vi "LabscanV1.vi"() -> ()   [LabVIEW 2019]
doc: "Ce Vi est le programme principale du système de spectroscopie pompe-sonde. Il permet d'effectuer des séries de mesures où l'on fait varier le délais entre un faisceaux d'excitation dit pompe et un faisceaux de mesure dit sonde, et où l'on mesure l'interaction des deux faisceaux en coupant momentanément le faisceau pompe. Le programme coordonne la ligne à délai, le shutter de la pompe et effectue l'acquisition de donnée. Les données sont affichées sur la fenêtres graphiques et on peut les sauvegarder dans un fichier texte. De multiple options sont disponible pour modifier les paramètres d'exécutions des balayages. Le programme facilite ainsi les mesures expérimentales."
uses:
  Experiment Class/Experiment.lvclass
  Interface Class/Interface.lvclass
  DevicesClass/BaseDevice/BaseDevice.lvclass
  <vilib>/Utility/miscctls.llb/LVPointTypeDef.ctl
  <vilib>/Utility/error.llb/DialogType.ctl
  <vilib>/event_ctls.llb/sizeaction.ctl
  <vilib>/event_ctls.llb/panelstate.ctl
  Interface Class/PlotChange.ctl
  <userlib>/GenProg/SetCtrlPropGen.vi
  Interface Class/Accessor/SetExperimentClass.vi
  <vilib>/Platform/browser.llb/Open URL in Default Browser (path).vi
  <userlib>/GenProg/SetCtrlPropGenSgl.vi
  DevicesClass/InstrumentsClass/MultiHarp150/MultiHarp150.lvclass
  DevicesClass/InstrumentsClass/AttoAMC/AttoAMC.lvclass
  DevicesClass/InstrumentsClass/TaikoLaser/TaikoLaser.lvclass
  DevicesClass/InstrumentsClass/ThorPM100A/ThorPM100A.lvclass
  DevicesClass/InstrumentsClass/AppliedMotionDrive/AppliedMotionDrive.lvclass
  DevicesClass/InstrumentsClass/ESP301/ESP301.lvclass
  DevicesClass/InstrumentsClass/AndorSpectro/AndorSpectro.lvclass
panel:
  in  "Load startup Exp.":bool=TRUE
  in  "Discard":bool
  in  "refresh test":bool
  out "Experiment Path":path
  out "queue out":refnum<queue>
  out "user event out":refnum<user-event>
  out "WrtGrpDel":u32
  out "WrtDatDel":u32
  in  "BaseDevice.lvclass":refnum<class "BaseDevice.lvclass">
  out "sem1":T1
  in  "DataFileRef":refnum<file>
  out "Exper.lvclass":refnum<class "Experiment.lvclass">
  out "ErrorOutAcq":errorcluster
  in  "HdrFileName":path
  out "error out":errorcluster
  in  "Error in":errorcluster
  out "ScanList":string[](array[string])
  in  "AcqEnd":bool caption="Fin Balayage"
  out "AcqComp":bool
  in  "Pause":bool
  in  "AcqStop":bool caption="Arrêt Balayage"
  out "Graph_VIs":refnum<vi>[](array[refnum])
  out "Graph_FA":refnum<vi>[](array[refnum])
  in  "stop":bool
  in  "Interface.lvclass":refnum<class "Interface.lvclass">
  in  "CtrlsTab":enum32{"Balayage", "Experiment", "Tracés"}(tab)
  in  "Single Par":bool caption="Single Parameter"
  in  "Scan Function":u16(ring) items=["Scan Pos (Arb)@Tools", "Indice de Point (Points)@Tools", "Scan Pos (Arb)@Tools_2", "Scan Pos (Arb)@Tools_3"]
  in  "path":path caption="Chemin du fichier de Sauvegarde"
  in  "Ouvrir":bool
  out "Temps Balayage":dbl format="%<%H:%M:%S>t"
  in  "DescKword":string caption="Description Keyword"
  in  "ScanFunc":string(tree) caption="Scan Functions"
  in  "MeasFunc":i32(listbox) caption="Measurements Instruments"
  out "MeasTime":u32 caption="Last Meas. Time (ms, all devices)"
  out "AvgPointTime(ms)":u32
  out "MeasTimes":u32[](array[numeric]) caption="Measurement Times (ms, by device)"
  out "ScanTimes":u32[](array[numeric]) caption="Scan Times (ms, by device)"
  in  "nb pos":i32 caption="Total Scan Points"
  out "Points Left":u32
  in  "Listbox":i32[](listbox)=[0] caption="Affichage des courbes"
  in  "Acq":bool caption="Balayage"
  # "Variables internes Balayages"
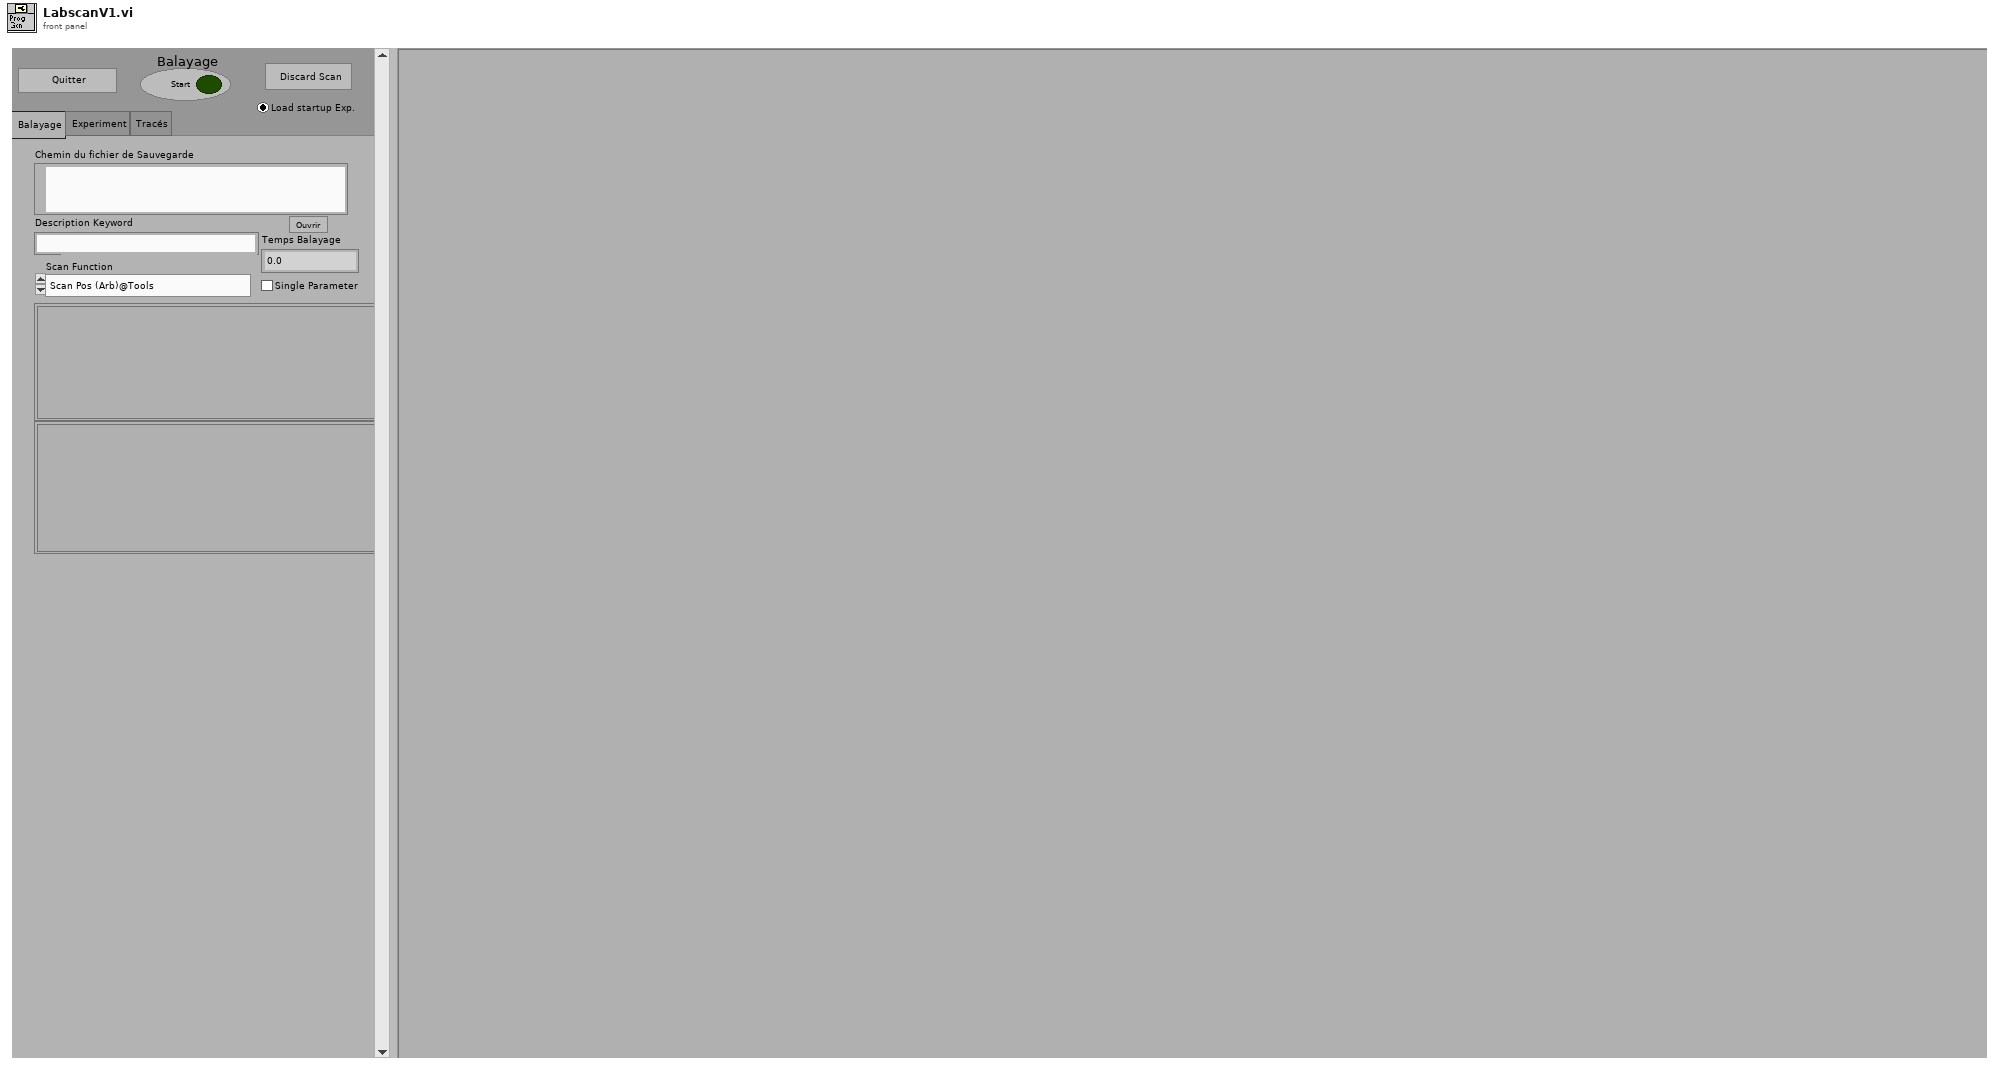
[diagram p1: front panel]
types:
  T1 = typedef "Semaphore RefNum" = refnum<k1>
  T2 = enum16{"Enable", "Disable", "DisAndGrayed", "ReinitToDefVal", "EnumElementsArr"}
  T3 = typedef "LVPointTypeDef.ctl" = cluster{"Horizontal":i16, "Vertical":i16}
  T4 = enum32{"Invalid", "Standard", "Closed", "Hidden", "Minimized", "Maximized"}
  T5 = enum16{"Répertoire du VI actuel", "Répertoire du parent 1", "Répertoire du parent 2", "Répertoire du parent 3"}
  T6 = enum16{"Text", "Background", "Item Symbol", "Open/Close Symbol", "Hierarchy Lines", "Right Border", "Bottom Border", "Bottom Right Corner", "Unknown Part"}
  T7 = typedef "panelstate.ctl" = enum32{"Standard", "Minimized", "Maximized"}
  T8 = typedef "sizeaction.ctl" = enum32{"Minimized", "Maximized", "Resized"}
  T9 = cluster{"Message":string, "Data":variant, "Code":i32}
  T10 = enum16{"No Item Sel", "One Item Sel", "Many Items Sel"}
  T11 = typedef "PlotChange.ctl" = cluster{"PlotIdx":i32, "PlotAttrib":cluster{"Color":u32, "PointStyle":u8, "LineStyle":u8, "Interp":u8, "LineWidth":u8, "BarPlotStyle":u8, "FillTo":i16, "XScaleIdx":u32, "YScaleIdx":u32, "Anti-Aliased":bool, "LabelFormat":u8, "TransitionType":u8, "TransitionLocation":u8, "DigitalLineStyle":u8}, "GraphId":i32, "Crv Visible":bool}
  T12 = cluster{dbl[], "XparInstrInd":i32, "YparInstrInd":i32}
  T13 = typedef "LVPositionTypeDef.ctl" = cluster{"Left":i32, "Top":i32}
  T14 = typedef "LVRectTypeDef.ctl" = cluster{"Left":i16, "Top":i16, "Right":i16, "Bottom":i16}
  T15 = typedef "DialogType.ctl" = u16
  T16 = typedef "Interface.lvclass/CurveSetup.ctl" = cluster{"CurveName":string, "YParam":string, "XParam":string, "ZParam ":string, "GroupName":string, "LinWdth":u8, "PntCol":u32, "LinCol":u32, "LablFor":u8, "XScale":u32, "YScale":u32, "Interpol":u8, "DisplayName":string, "FillType":i16, "LineStyle":u8, "PntStyle":u8, "BarTyp":u8, "GraphIndex":i32, "Visible":bool, "XScaleName":string, "YScaleName":string, "XYGraph_Ref":refnum<vi>, "Data Only":bool, "DataQ Ref":refnum<queue>, "XParQ Ref":refnum<queue>, "XParamInd":i32, "ScanInd":i32, "File Path":path}
  T17 = typedef "ArrDevData.ctl" = cluster{"MeasDatOut":dbl[][], "XDatOut":dbl[][], "YDatOut":dbl[][], "DevID":i32}
  T18 = enum16{"Left Button", "Center Button", "Right Button", "Window Close"}
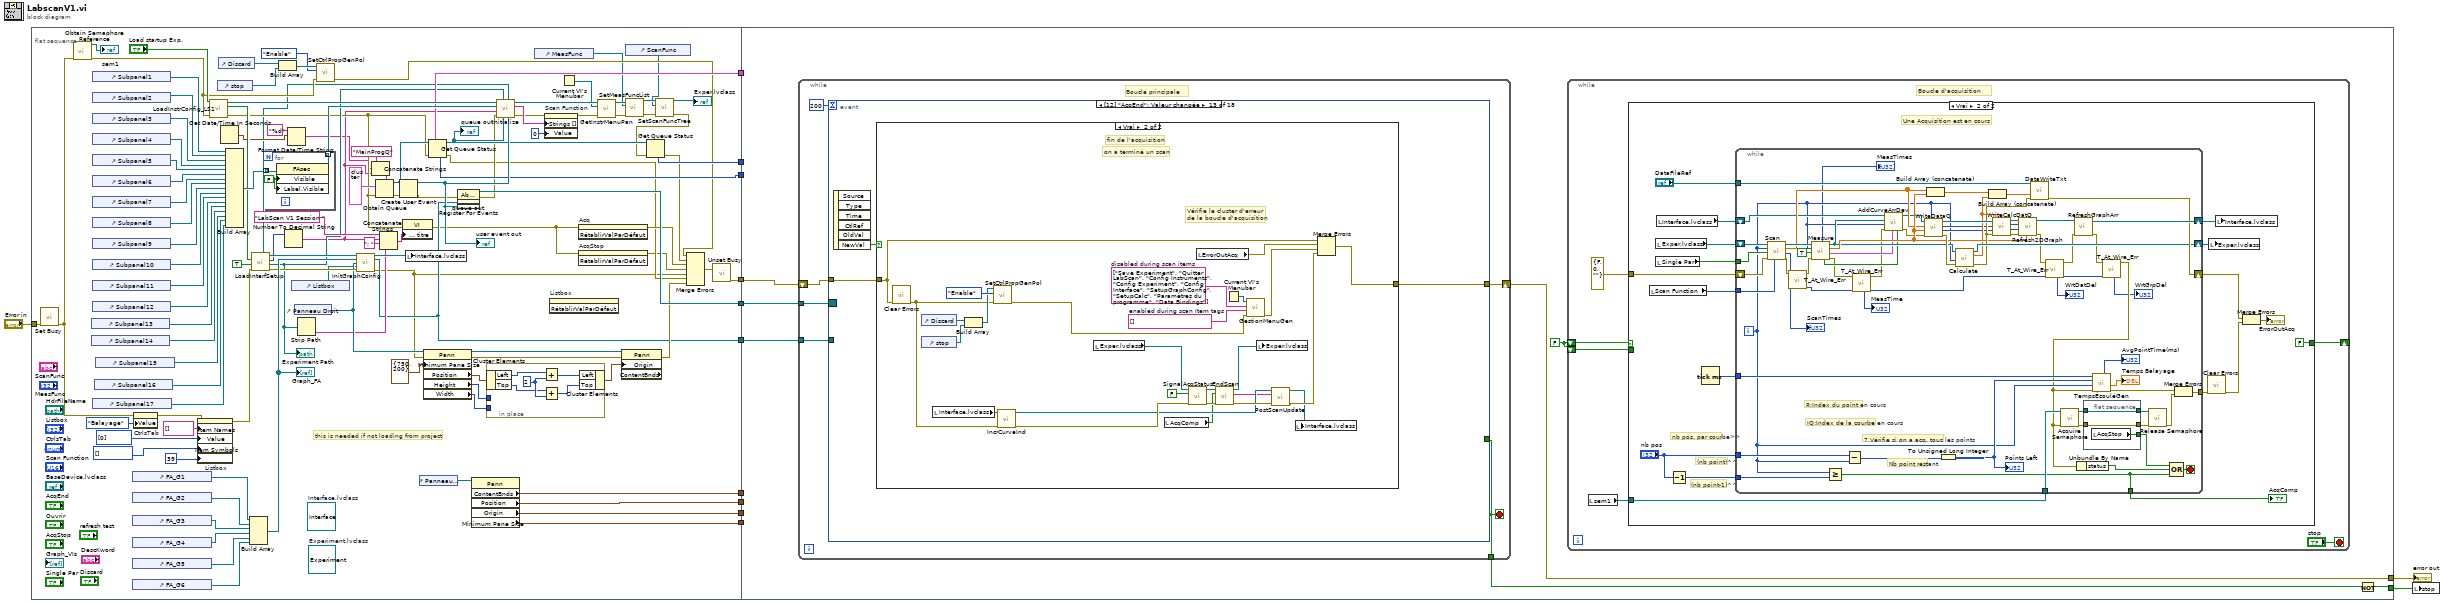
[diagram p0: block diagram]
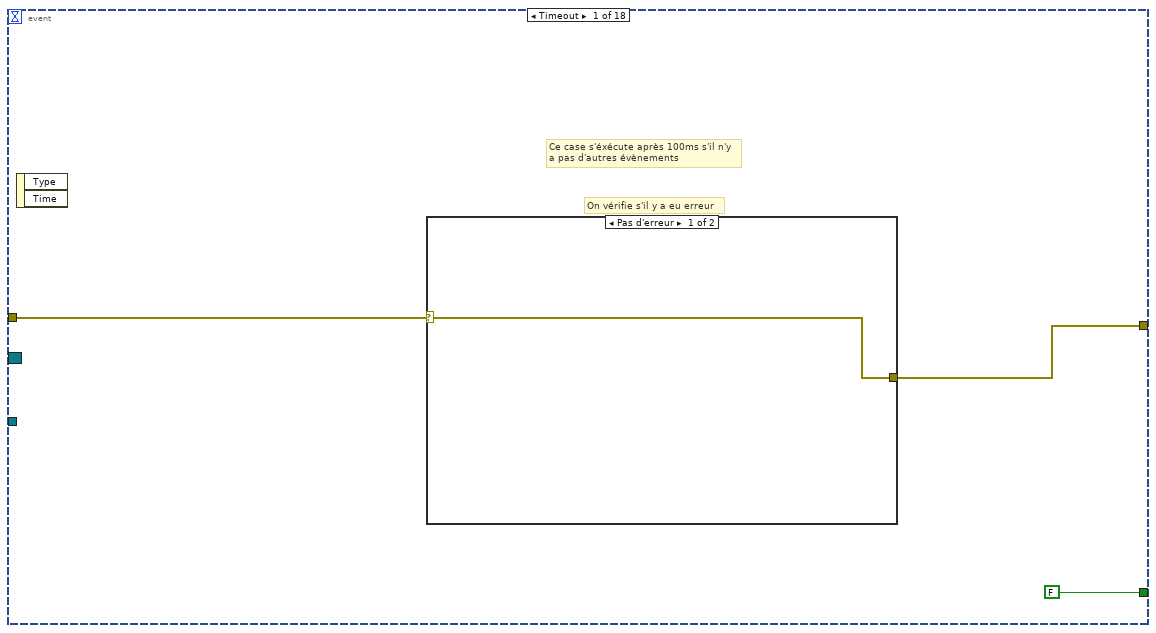
[diagram p2: hidden frame]
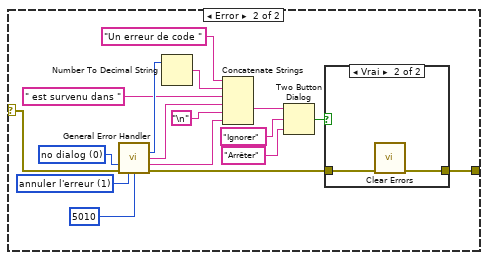
[diagram p3: hidden frame]
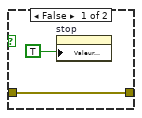
[diagram p4: hidden frame]
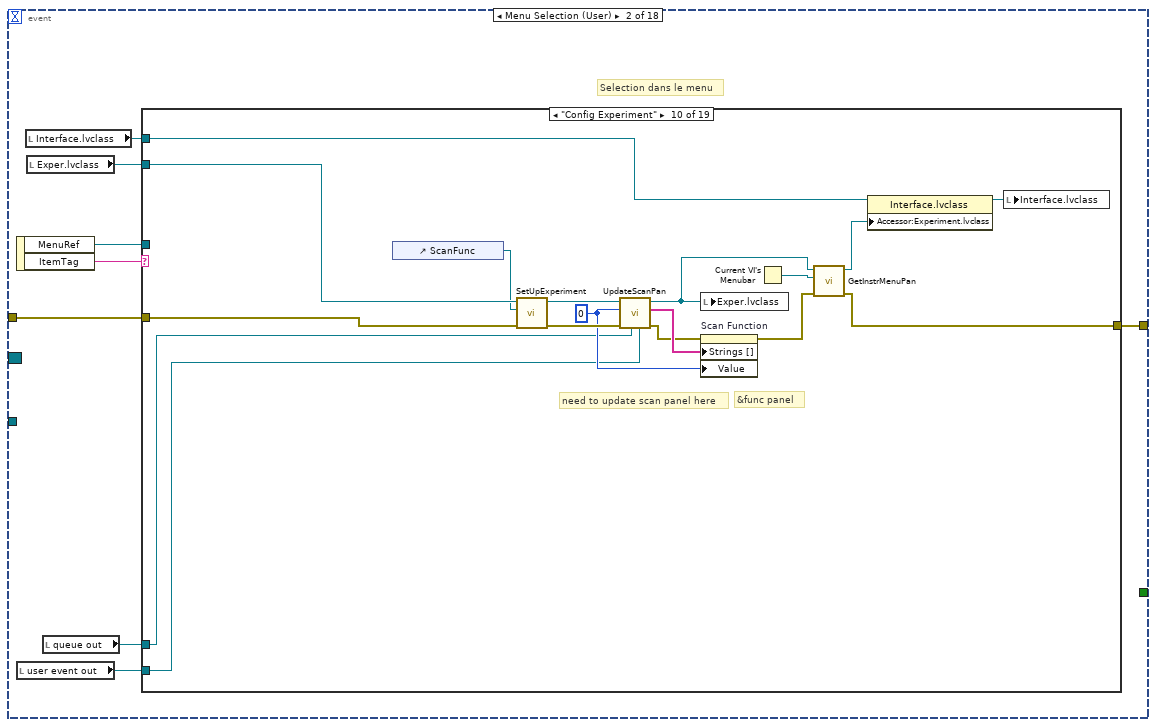
[diagram p5: hidden frame]
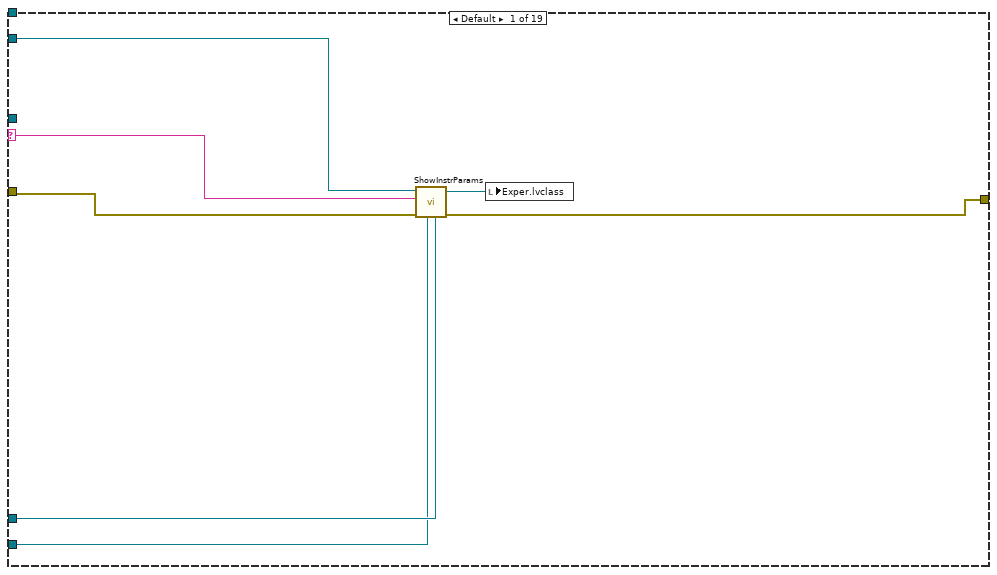
[diagram p6: hidden frame]
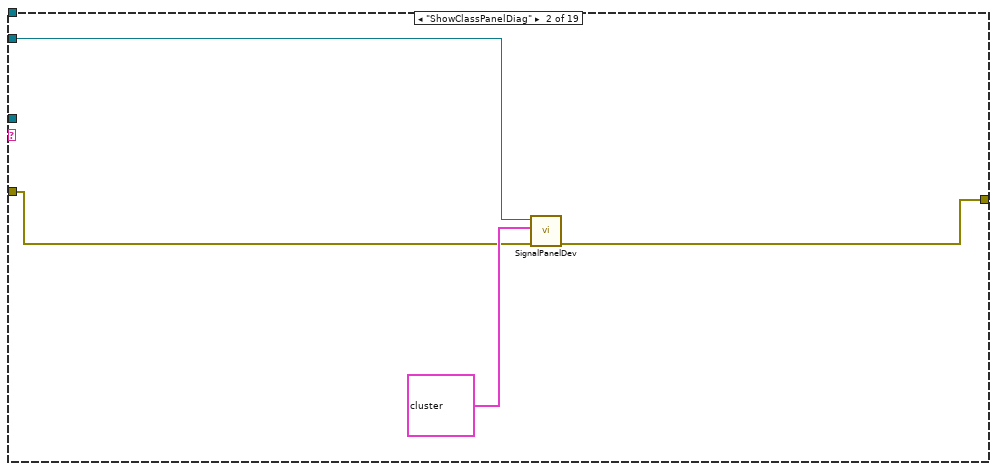
[diagram p7: hidden frame]
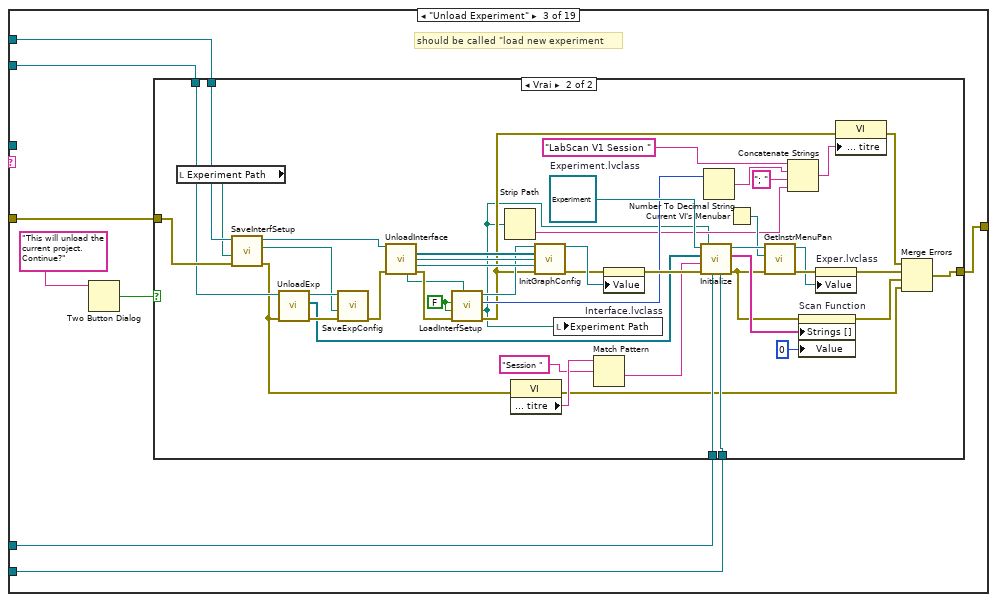
[diagram p8: hidden frame]
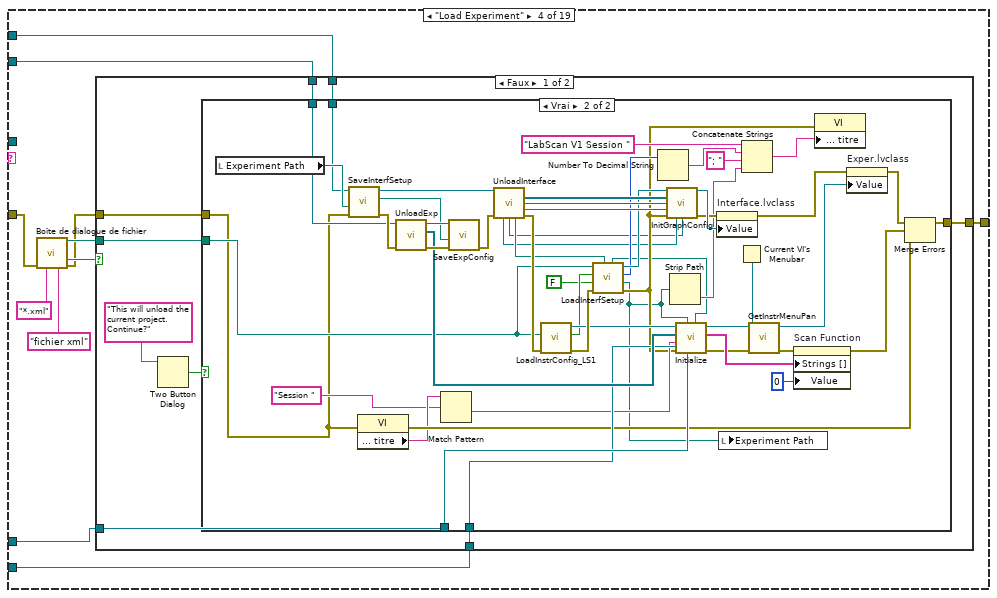
[diagram p10: hidden frame]
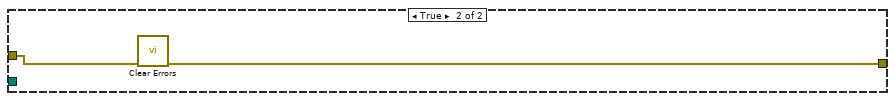
[diagram p12: hidden frame]
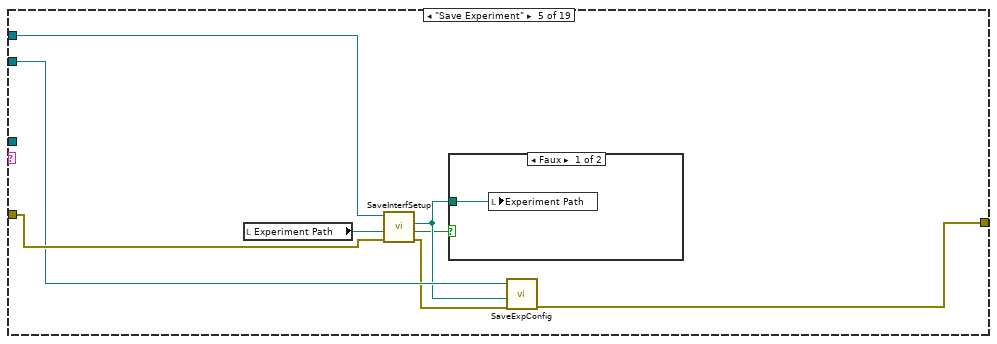
[diagram p13: hidden frame]
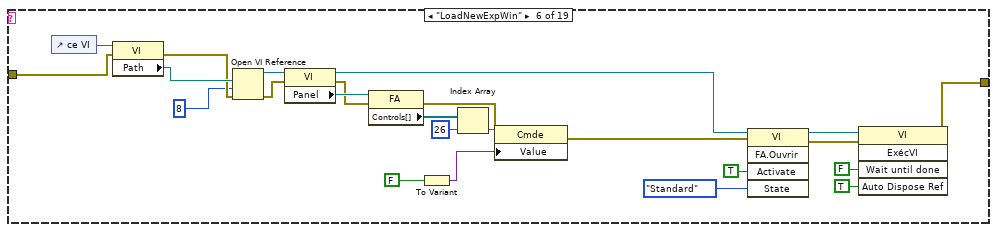
[diagram p15: hidden frame]
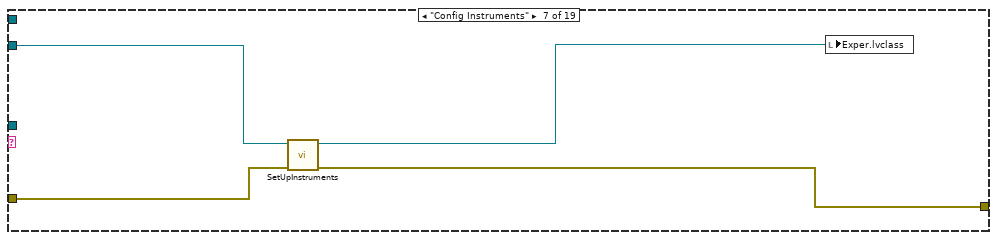
[diagram p16: hidden frame]
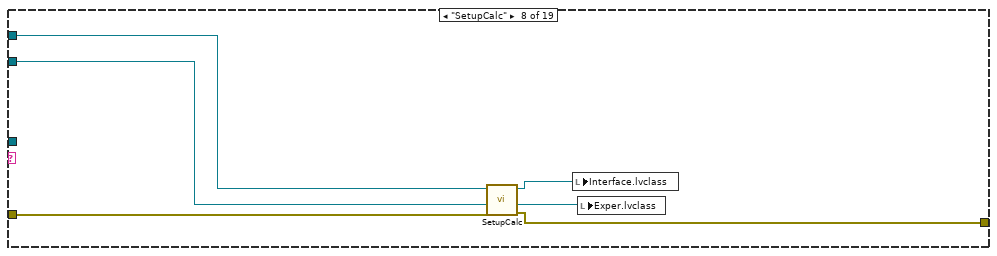
[diagram p17: hidden frame]
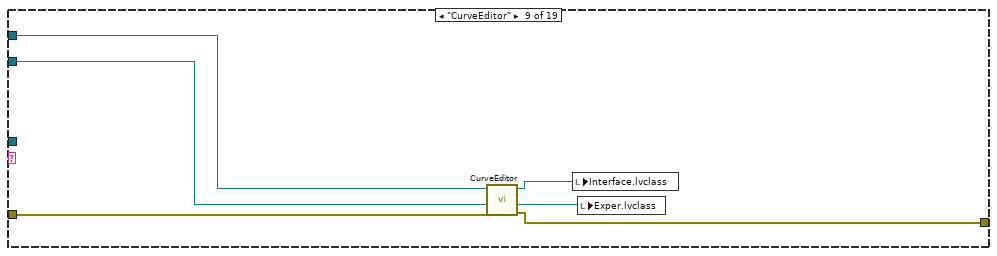
[diagram p18: hidden frame]
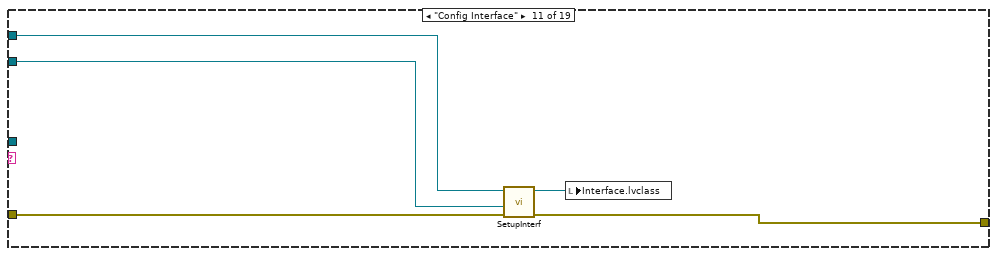
[diagram p19: hidden frame]
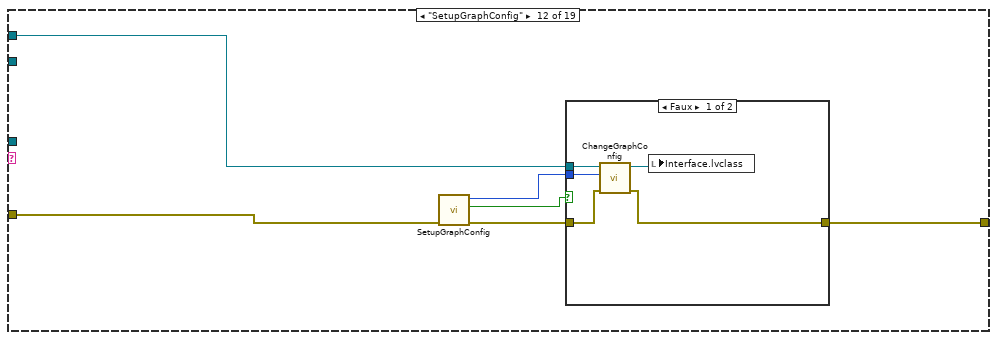
[diagram p20: hidden frame]
diagram:
  n1 = flat-sequence {
    tunnel: "Error in" -> [w121]
    tunnel: [w122] -> w11
    tunnel: [w100] -> w9
    tunnel: [w93] -> w8
    tunnel: [w94] -> w7
    tunnel: [w84] -> w6
    tunnel: [w82] -> w5
    tunnel: [w67] -> w4
    tunnel: [w66] -> w3
    tunnel: [w65] -> w2
    tunnel: [w63] -> w1
    tunnel: [w138] -> w10
    tunnel: [w136] -> w13
    tunnel: w11 -> [w134]
    tunnel: w9 -> [_]
    tunnel: w8 -> [_]
    tunnel: w7 -> [_]
    tunnel: w6 -> [w135]
    tunnel: w5 -> [_]
    tunnel: w4 -> [_]
    tunnel: w3 -> [_]
    tunnel: w2 -> [w133]
    tunnel: w1 -> [_]
    frame #0 {
      (unwired) refnum<class "Interface.lvclass"> refnum  # Interface.lvclass
      (unwired) refnum<class "Experiment.lvclass"> refnum  # Experiment.lvclass
      # "this is needed if not loading from project"
      n2 = call <vilib>:"Set Busy.vi"("error in (no error)"=w121) -> ("error out"=w54:errorcluster)  [unwired: 9 in, 1 out]
      n3 = call <vilib>:"Obtain Semaphore Reference.vi"("error in (no error)"=w54) -> ("error out"=w42:errorcluster, "semaphore"=→"sem1":T1)  [unwired: 4 in, 1 out]
      n4 = control-ref of="Subpanel13"() -> (w27:refnum<vi>)
      n5 = control-ref of="Subpanel14"() -> (w26:refnum<vi>)
      n6 = control-ref of="Subpanel1"() -> (w115:refnum<vi>)
      n7 = control-ref of="Subpanel2"() -> (w33:refnum<vi>)
      n8 = control-ref of="Subpanel3"() -> (w120:refnum<vi>)
      n9 = control-ref of="Subpanel4"() -> (w119:refnum<vi>)
      n10 = control-ref of="Subpanel5"() -> (w77:refnum<vi>)
      n11 = control-ref of="Subpanel6"() -> (w52:refnum<vi>)
      n12 = control-ref of="Subpanel7"() -> (w40:refnum<vi>)
      n13 = control-ref of="Subpanel8"() -> (w31:refnum<vi>)
      n14 = control-ref of="Subpanel9"() -> (w30:refnum<vi>)
      n15 = control-ref of="Subpanel10"() -> (w32:refnum<vi>)
      n16 = control-ref of="Subpanel11"() -> (w29:refnum<vi>)
      n17 = control-ref of="Subpanel12"() -> (w28:refnum<vi>)
      n18 = control-ref of="Subpanel17"() -> (w14:refnum<vi>)
      n19 = control-ref of="Subpanel16"() -> (w15:refnum<vi>)
      n20 = control-ref of="Subpanel15"() -> (w16:refnum<vi>)
      n21 = control-ref of="FA_G1"() -> (w107:refnum<vi>)
      n22 = control-ref of="FA_G2"() -> (w112:refnum<vi>)
      n23 = control-ref of="FA_G3"() -> (w111:refnum<vi>)
      n24 = control-ref of="FA_G4"() -> (w110:refnum<vi>)
      n25 = control-ref of="FA_G5"() -> (w109:refnum<vi>)
      n26 = control-ref of="FA_G6"() -> (w108:refnum<vi>)
      n27 = property on="CtrlsTab" class="Onglet (strict)"(error in=w54, "Value"=enum32{"Balayage", "Experiment", "Tracés"}."Balayage" ("CtrlsTab")) -> (error out=w92:errorcluster)  [unwired: 1 in, 1 out]
      n28 = property on="Listbox" class="LstDér (strict)"(error in=w92, "Item Names"=string[] [] ("Noms d'éléments"), "Value"=i32[] [0] ("Listbox"), "Item Symbols"=i32[] [] ("Listbox"), "Number of Rows"=39 ("Ligne en focus")) -> (error out=w44:errorcluster)  [unwired: 1 in, 1 out]
      n29 = call "LoadInstrConfig_LS1.vi"("error in (no error)"=w42, "LoadExp"="Load startup Exp.") -> ("error out"=w41:errorcluster, "LoadExper Out"=w88:bool, "Experiment.lvclass"=w117:refnum<class "Experiment.lvclass">)  [unwired: 6 in, 1 out]
      n30 = control-ref of="stop"() -> (w58:refnum<vi>)
      n31 = control-ref of="Discard"() -> (w56:refnum<vi>)
      n32 = Get Date/Time In Seconds() -> (seconds since 1Jan1904=w36:timestamp)
      n33 = Build Array(w115, w33, w120, w119, w77, w52, w40, w31, w30, w32, w29, w28, w27, w26, w16, w15, w14) -> (w118:refnum<vi>[])
      n34 = Build Array(w107, w112, w111, w110, w109, w108) -> (w105:refnum<vi>[])
      "Graph_FA" <- w105
      n35 = call "LoadInterfSetup.vi"("ErrIn (NoErr)"=w44, "IncrSession"=TRUE, "LoadIntf?"=w88) -> ("error out"=w104:errorcluster, "Experiment Path"=w43:path, "Session"=w79:i32, "Interface en sortie"=w103:refnum<class "Interface.lvclass">, "BaseDataPath out"=w34:path)  [unwired: 4 in]
      "Experiment Path" <- w43
      n36 = for {
        tunnel: w118 -> [w132] mode=indexing
        tunnel: [w131] -> w90 mode=indexing
        w130 = FALSE ("Visible")
        n37 = property class="FAsec"(reference=w132, "Visible"=w130, "Label.Visible"=w130) -> (reference out=w131:refnum<vi>)  [unwired: 1 in, 1 out]
      }
      n38 = Build Array(w56, w58) -> (w57:refnum<vi>[])
      n39 = Number To Decimal String(number=w79) -> (decimal integer string=w38:string)  [unwired: 1 in]
      n40 = Format Date/Time String(time format string (%c)="%d" ("chaîne de format de l'heure (%c)"), seconds (now)=w36) -> (date/time string=w35:string)  [unwired: 1 in]
      n41 = control-ref of="Listbox"() -> (w49:refnum<vi>)
      n42 = control-ref of="Panneau Droit"() -> (w99:refnum<vi>)
      n43 = Strip Path(path=w43) -> (name=w68:string)  [unwired: 1 out]
      n44 = call-poly <userlib>:"SetCtrlPropGenPol.vi"("Error in"=w42, "Énum"=T2."Enable", "Controls"=w57) -> ("Error out"=w53:errorcluster)  [unwired: 3 in, 1 out]
      n45 = call "InitGraphConfig.vi"("Interface en entrée"=w103, "Graph_FA"=w105, "PanRef"=w99, "ListboxRef"=w49, "error in (no error)"=w104) -> ("Interface en sortie"=w102:refnum<class "Interface.lvclass">, "Graph Event"=w65:refnum<user-event>, "error out"=w48:errorcluster)  [unwired: 8 in]
      n46 = Concatenate Strings("MainProgQ" ("nom (aucun)"), w35, w38) -> (w39:string)
      n47 = Obtain Queue(name (unnamed)=w39, element data type=cluster{"Message":string, "Data":variant, i32} {"Message"="", "Data"=variant, 0} ("ClassQueue"), error in (no error)=w41) -> (queue out=w72:refnum<queue>, error out=w76:errorcluster)  [unwired: 2 in, 1 out]
      n48 = Concatenate Strings("LabScan V1 Session " ("Front Panel Window:Title"), w38, "; " ("string"), w68) -> (w61:string)
      n49 = Create User Event(user event datatype=w72, error in=w76) -> (user event=w73:refnum<user-event>, error out=w62:errorcluster)
      "user event out" <- w73
      n50 = property class="VI"(error in=w41, "Fenêtre face-avant : titre"=w61) -> (error out=w51:errorcluster)  [unwired: 1 in, 1 out]
      n51 = local write "Interface.lvclass"(w102) -> ()
      n52 = control-ref of="Panneau Gauche"() -> (w101:refnum<vi>)
      n53 = property class="Pann"(reference=w99, error in=w48, "Minimum Pane Size"=T3 {"Horizontal"=750, "Vertical"=200} ("Taille minimale de panneau")) -> (reference out=w97:refnum<vi>, error out=w89:errorcluster, "Position"=w96:T13, "Height"=w81:u32, "Width"=w80:u32)
      n54 = Get Queue Status(queue=w72, error in (no error)=w41) -> (queue out=w64:refnum<queue>, error out=w59:errorcluster, # elements in queue=w67:i32, elements=w66:cluster{"Message":string, "Data":variant, i32}[])  [unwired: 1 in, 4 out]
      "queue out" <- w64
      n55 = register-events(error in=w62, w65, w73) -> (reference out=w84:refnum<event-registration>, error out=w60:errorcluster)  [unwired: 1 in]
      n56 = property class="Pann"(reference=w101) -> ("ContentBnds"=w100:T14, "Position"=w93:T13, "Origin"=w94:T3, "Minimum Pane Size"=w82:T3)  [unwired: 1 in, 2 out]
      n57 = in-place {
        in-place-border: w81 -> [_]
        in-place-border: w80 -> [_]
        w127 = 2 ("y")
        n58 = in-place-cluster #1(w96) -> ("Left"=w129:i32, "Top"=w126:i32)
        n59 = Add(x=w129, y=w127) -> (x+y=w128:i32)
        n60 = Add(x=w126, y=w127) -> (x+y=w125:i32)
        n61 = in-place-cluster #1("Left"=w128, "Top"=w125) -> (w95:T13)
      }
      n62 = call "Initialize.vi"("MainProgQEvent"=w73, "BaseDataPath"=w34, "MainProgQ"=w64, "Experiment Path"=w43, "ErrIn (NoErr)"=w60, "Session"=w38, "SubPanel Refs"=w90, "Experiment In"=w117) -> ("error out"=w114:errorcluster, "PanScanFunc"=w116:string[], "Experiment Out"=w87:refnum<class "Experiment.lvclass">)  [unwired: 1 in]
      n63 = control-ref of="MeasFunc"() -> (w23:refnum<vi>)
      n64 = property on="Scan Function" class="MDér (strict)"(error in=w114, "Strings []"=w116, "Value"=0) -> (error out=w86:errorcluster)  [unwired: 1 in, 1 out]
      n65 = invoke on="Listbox" class="LstDér (strict)" method="RétablirValParDéfaut"() -> ()  [unwired: 3 in, 3 out]
      n66 = Current VI's Menubar() -> (w85:refnum<k9>)
      n67 = invoke on="Acq" class="Bool (strict)" method="RétablirValParDéfaut"(error in=w51) -> (error out=w70:errorcluster)  [unwired: 2 in, 2 out]
      n68 = invoke on="AcqStop" class="Bool (strict)" method="RétablirValParDéfaut"(error in=w51) -> (error out=w50:errorcluster)  [unwired: 2 in, 2 out]
      n69 = call "GetInstrMenuPan.vi"("error in (no error)"=w86, "référence de menu"=w85, "Experiment en entrée"=w87) -> ("error out"=w25:errorcluster, "Experiment en sortie"=w24:refnum<class "Experiment.lvclass">)  [unwired: 7 in]
      n70 = property class="Pann" props=["Origin", "ContentBnds"](reference=w97, error in=w89, "Origin"=w95) -> (error out=w83:errorcluster)  [unwired: 2 out]
      n71 = call "SetMeasFuncList.vi"("error in (no error)"=w25, "ListRef"=w23, "Experiment en entrée"=w24) -> ("error out"=w18:errorcluster, "Experiment en sortie"=w21:refnum<class "Experiment.lvclass">)  [unwired: 7 in]
      n72 = control-ref of="ScanFunc"() -> (w19:refnum<vi>)
      n73 = call "SetScanFuncTree.vi"("error in (no error)"=w18, "ScanTreeRef"=w19, "Experiment en entrée"=w21) -> ("error out"=w17:errorcluster, "Experiment en sortie"=→"Exper.lvclass":refnum<class "Experiment.lvclass">)  [unwired: 7 in]
      n74 = Get Queue Status(queue=w64, error in (no error)=w17) -> (# elements in queue=w63:i32)  [unwired: 1 in, 7 out]
      n75 = Merge Errors(w53, w17, w70, w50, w48, w59, w83) -> (w123:errorcluster)
      n76 = call <vilib>:"Unset Busy.vi"("error in (no error)"=w123) -> ("error out"=w122:errorcluster)  [unwired: 10 in]
    }
    frame #1 {
      w137 = FALSE
      n77 = while {
        tunnel: [w142] -> w139
        shift-right: [w144] -> w138
        shift-left: w134 -> [w143]
        tunnel: w135 -> [w141]
        tunnel: w133 -> [w140]
        stop <- w142 stop-if-true
        # "Boucle principale"
        n78 = event shown="[12] \"AcqEnd\": Valeur changée" {
          selector: w141 -> [_ _ _ _ _ _ _ _ _ _ _ _ _ _ _ _ _ _]
          dyn-events: _ -> [_ _ _ _ _ _ _ _ _ _ _ _ _ _ _ _ _ _]
          timeout: 200 -> [_ _ _ _ _ _ _ _ _ _ _ _ _ _ _ _ _ _]
          tunnel: [w148 w177 w442 w463 w486 w507 w684 _ w795 w849 w955 w971 w1054 w1085 w1090 w1096 w1114 w1147] -> w144
          tunnel: w143 -> [w146 w176 w445 w464 w487 w508 w681 _ w800 w848 w956 w976 w1053 w1089 w1091 w1095 w1115 w1148]
          tunnel: [FALSE _ _ _ _ _ _ _ _ _ _ _ _ _ _ _ _ w1149] -> w142
          tunnel: w140 -> [_ _ _ _ _ _ w675 _ _ _ _ _ _ _ _ _ _ _]
          event Timeout {
            # "On vérifie s'il y a eu erreur"
            # "Ce case s'éxécute après 100ms s'il n'y a pas d'autres évènements"
            n79 = event-data() -> ()  [unwired: 1 in, 2 out]
            n80 = case shown="Pas d'erreur" w146 {
              selector: w146 -> [w149 w152]
              tunnel: [w149 w153] -> w148
              frame No Error {
              }
              frame Error {
                w151 = 1 items=["pas d'exception", "annuler l'erreur", "définir l'erreur"] ("[exception action] (none:0)")
                w163 = T15 0 items=["no dialog", "OK message", "continue or stop message", "OK message + warnings", "continue/stop + warnings"] ("type of dialog (OK msg:1)")
                n81 = call <vilib>:"General Error Handler.vi"("type of dialog (OK msg:1)"=w163, "error in (no error)"=w152, "[exception action] (none:0)"=w151, "[exception code]"=5010) -> ("code out"=w159:i32, "source out"=w158:string, "message"=w156:string, "error out"=w154:errorcluster)  [unwired: 7 in, 1 out]
                n82 = Number To Decimal String(number=w159) -> (decimal integer string=w160:string)  [unwired: 1 in]
                n83 = Concatenate Strings("Un erreur de code " ("string"), w160, " est survenu dans " ("string"), w158, "\n", w156) -> (w155:string)
                n84 = Two Button Dialog(message=w155, 1:"Arrêter" ("F button name (\"Cancel\")"), 2:"Ignorer" ("T button name (\"OK\")")) -> (T button?=w166:bool)
                n85 = case shown="Vrai" w166 {
                  tunnel: w154 -> [w168 w169]
                  tunnel: [w168 w170] -> w153
                  frame False {
                    n86 = property on="stop" class="Bool (strict)"("Valeur (Signalisation)"=TRUE ("Value (Signaling)")) -> ()  [unwired: 2 in, 2 out]
                  }
                  frame True {
                    n87 = call <vilib>:"Clear Errors.vi"("error in (no error)"=w169) -> ("error out"=w170:errorcluster)  [unwired: 5 in, 1 out]
                  }
                }
              }
            }
          }
          event Menu Selection (User) {
            # "Selection dans le menu"
            n88 = event-data() -> ("MenuRef"=w175:refnum<k9>, "ItemTag"=w178:string)  [unwired: 1 in]
            n89 = local read "user event out"() -> (w171:refnum<user-event>)
            n90 = local read "Interface.lvclass"() -> (w173:refnum<class "Interface.lvclass">)
            n91 = local read "Exper.lvclass"() -> (w174:refnum<class "Experiment.lvclass">)
            n92 = local read "queue out"() -> (w172:refnum<queue>)
            n93 = case shown="\"Config Experiment\"" w178 {
              selector: w178 -> [w181 _ _ _ _ _ _ _ _ _ _ _ _ _ _ _ _ _ _]
              tunnel: [w182 w187 w194 w254 w325 w346 w354 w362 w368 w371 w389 w395 w406 w419 w425 w428 w433 w437 w439] -> w177
              tunnel: w176 -> [w183 w188 w196 w247 w326 w350 w357 w363 w369 w386 w390 w397 w414 w420 w425 w430 w434 w438 w440]
              tunnel: w175 -> [_ _ _ _ _ _ _ _ _ _ _ _ _ _ _ _ _ _ _]
              tunnel: w174 -> [w185 w186 w195 w255 w324 _ w356 w361 w367 w385 w388 _ _ _ w423 w431 _ _ _]
              tunnel: w173 -> [_ _ w197 w256 w327 _ _ w360 w366 w379 w387 w393 w408 w418 w424 _ _ _ _]
              tunnel: w172 -> [w180 _ w191 w249 _ _ _ _ _ w374 _ _ w405 _ _ _ _ _ _]
              tunnel: w171 -> [w179 _ w190 w248 _ _ _ _ _ w373 _ _ w404 _ _ _ _ _ _]
              frame Default {
                n94 = call "ShowInstrParams.vi"("queue out"=w180, "user event out"=w179, "error in (no error)"=w183, "InstrParam"=w181, "Experiment en entrée"=w185) -> ("error out"=w182:errorcluster, "Experiment en sortie"=w184:refnum<class "Experiment.lvclass">)  [unwired: 5 in]
                n95 = local write "Exper.lvclass"(w184) -> ()
              }
              frame "ShowClassPanelDiag" {
                n96 = call "SignalPanelDev.vi"("error in (no error)"=w188, "Message"=cluster{"Message":string, "Data":variant, i32} {"Message"="ShowDiag", "Data"=variant, 0}, "Experiment en entrée"=w186) -> ("error out"=w187:errorcluster)  [unwired: 7 in, 1 out]
              }
              frame "Unload Experiment" {
                # "should be called \"load new experiment"
                n97 = Two Button Dialog(message="This will unload the current project. Continue?") -> (T button?=w192:bool)  [unwired: 2 in]
                n98 = case shown="Vrai" w192 {
                  tunnel: w197 -> [_ w240]
                  tunnel: w196 -> [w198 w239]
                  tunnel: w195 -> [_ w238]
                  tunnel: [w198 w223] -> w194
                  tunnel: w191 -> [_ w216]
                  tunnel: w190 -> [_ w215]
                  frame False {
                  }
                  frame True {
                    w214 = FALSE ("LoadIntf?")
                    w229 = refnum<class "Experiment.lvclass"> refnum  # Experiment.lvclass
                    n99 = local read "Experiment Path"() -> (w208:path)
                    n100 = call "SaveInterfSetup.vi"("error in (no error)"=w239, "Experiment Path"=w208, "Interface en entrée"=w240) -> ("error out"=w211:errorcluster, "SavePath"=w241:path, "Interface en sortie"=w243:refnum<class "Interface.lvclass">)  [unwired: 5 in, 1 out]
                    n101 = call "UnloadExp.vi"("error in (no error)"=w211, "Experiment en entrée"=w238) -> ("error out"=w244:errorcluster, "SubpanelRefs"=w230:refnum<vi>[], "Experiment en sortie"=w245:refnum<class "Experiment.lvclass">)  [unwired: 7 in]
                    n102 = call "SaveExpConfig.vi"("error in (no error)"=w244, "Experiment"=w241, "Experiment.lvclass"=w245) -> ("error out"=w242:errorcluster)  [unwired: 7 in, 1 out]
                    n103 = call "UnloadInterface.vi"("Interface en entrée"=w243, "error in (no error)"=w242) -> ("Graph_FA"=w234:refnum<vi>[], "PanRef"=w235:refnum<vi>, "ListBoxRef"=w236:refnum<vi>, "BaseDataPath"=w226:path, "error out"=w227:errorcluster)  [unwired: 6 in, 3 out]
                    n104 = call "LoadInterfSetup.vi"("BaseDataPath"=w226, "ErrIn (NoErr)"=w227, "IncrSession"=w214, "LoadIntf?"=w214) -> ("error out"=w200:errorcluster, "Experiment Path"=w199:path, "Session"=w203:i32, "Interface en sortie"=w228:refnum<class "Interface.lvclass">)  [unwired: 3 in, 1 out]
                    n105 = Strip Path(path=w199) -> (name=w202:string)  [unwired: 1 out]
                    n106 = property class="VI"(error in=w211) -> (error out=w209:errorcluster, "Fenêtre face-avant : titre"=w213:string)  [unwired: 1 in, 1 out]
                    n107 = call "InitGraphConfig.vi"("Interface en entrée"=w228, "Graph_FA"=w234, "PanRef"=w235, "ListboxRef"=w236, "error in (no error)"=w200) -> ("Interface en sortie"=w233:refnum<class "Interface.lvclass">, "error out"=w232:errorcluster)  [unwired: 8 in, 1 out]
                    n108 = local write "Experiment Path"(w199) -> ()
                    n109 = Match Pattern(string=w213, regular expression="Session ") -> (after substring=w210:string)  [unwired: 1 in, 3 out]
                    n110 = property on="Interface.lvclass" class="CmdeClasseLV (strict)"(error in=w232, "Value"=w233) -> (error out=w231:errorcluster)  [unwired: 1 in, 1 out]
                    n111 = call "Initialize.vi"("MainProgQEvent"=w215, "MainProgQ"=w216, "Experiment Path"=w199, "ErrIn (NoErr)"=w231, "Session"=w210, "SubPanel Refs"=w230, "Experiment In"=w229) -> ("error out"=w220:errorcluster, "PanScanFunc"=w224:string[], "Experiment Out"=w219:refnum<class "Experiment.lvclass">)  [unwired: 2 in]
                    n112 = Number To Decimal String(number=w203) -> (decimal integer string=w204:string)  [unwired: 1 in]
                    n113 = Current VI's Menubar() -> (w217:refnum<k9>)
                    n114 = call "GetInstrMenuPan.vi"("error in (no error)"=w220, "référence de menu"=w217, "Experiment en entrée"=w219) -> ("error out"=w221:errorcluster, "Experiment en sortie"=w218:refnum<class "Experiment.lvclass">)  [unwired: 7 in]
                    n115 = Concatenate Strings("LabScan V1 Session " ("Front Panel Window:Title"), w204, "; " ("string"), w202) -> (w207:string)
                    n116 = property on="Scan Function" class="MDér (strict)"(error in=w220, "Strings []"=w224, "Value"=0) -> (error out=w222:errorcluster)  [unwired: 1 in, 1 out]
                    n117 = property on="Exper.lvclass" class="CmdeClasseLV (strict)"(error in=w221, "Value"=w218) -> (error out=w237:errorcluster)  [unwired: 1 in, 1 out]
                    n118 = property class="VI"(error in=w200, "Fenêtre face-avant : titre"=w207) -> (error out=w201:errorcluster)  [unwired: 1 in, 1 out]
                    n119 = Merge Errors(w201, w237, w222, w209) -> (w223:errorcluster)
                  }
                }
              }
              frame "Load Experiment" {
                n120 = call "Boîte de dialogue de fichier"("error in"=w247, "pattern (all files)"="*.xml", "pattern label"="fichier xml") -> ("selected path"=w250:path, "cancelled"=w251:bool, "error out"=w246:errorcluster)  [unwired: 9 in, 1 out]
                n121 = case shown="Faux" w251 {
                  tunnel: w256 -> [w265 _]
                  tunnel: w246 -> [w264 w320]
                  tunnel: w255 -> [w263 _]
                  tunnel: [w262 w319] -> w254
                  tunnel: w250 -> [w259 _]
                  tunnel: w249 -> [w258 _]
                  tunnel: w248 -> [w257 _]
                  frame False {
                    n122 = Two Button Dialog(message="This will unload the current project. Continue?") -> (T button?=w261:bool)  [unwired: 2 in]
                    n123 = case shown="Vrai" w261 {
                      tunnel: w265 -> [_ w271]
                      tunnel: w264 -> [w266 w279]
                      tunnel: w263 -> [_ w312]
                      tunnel: [w266 w296] -> w262
                      tunnel: w259 -> [_ w280]
                      tunnel: w258 -> [_ w288]
                      tunnel: w257 -> [_ w287]
                      frame False {
                      }
                      frame True {
                        n124 = local read "Experiment Path"() -> (w281:path)
                        n125 = call "SaveInterfSetup.vi"("error in (no error)"=w279, "Experiment Path"=w281, "Interface en entrée"=w271) -> ("error out"=w315:errorcluster, "SavePath"=w313:path, "Interface en sortie"=w316:refnum<class "Interface.lvclass">)  [unwired: 5 in, 1 out]
                        n126 = property class="VI"(error in=w279) -> (error out=w285:errorcluster, "Fenêtre face-avant : titre"=w284:string)  [unwired: 1 in, 1 out]
                        n127 = call "UnloadExp.vi"("error in (no error)"=w315, "Experiment en entrée"=w312) -> ("error out"=w317:errorcluster, "SubpanelRefs"=w305:refnum<vi>[], "Experiment en sortie"=w318:refnum<class "Experiment.lvclass">)  [unwired: 7 in]
                        n128 = Match Pattern(string=w284, regular expression="Session ") -> (after substring=w282:string)  [unwired: 1 in, 3 out]
                        n129 = call "SaveExpConfig.vi"("error in (no error)"=w317, "Experiment"=w313, "Experiment.lvclass"=w318) -> ("error out"=w314:errorcluster)  [unwired: 7 in, 1 out]
                        n130 = call "UnloadInterface.vi"("Interface en entrée"=w316, "error in (no error)"=w314) -> ("Graph_FA"=w308:refnum<vi>[], "PanRef"=w309:refnum<vi>, "ListBoxRef"=w310:refnum<vi>, "GraphEvent"=w270:refnum<user-event>, "MainGraphQ"=w269:refnum<queue>, "BaseDataPath"=w299:path, "error out"=w303:errorcluster)  [unwired: 6 in, 1 out]
                        n131 = call "LoadInstrConfig_LS1.vi"("error in (no error)"=w303, "Experiment"=w280) -> ("error out"=w302:errorcluster, "LoadExper Out"=w300:bool, "Experiment.lvclass"=w301:refnum<class "Experiment.lvclass">)  [unwired: 6 in, 1 out]
                        n132 = call "LoadInterfSetup.vi"("BaseDataPath"=w299, "ErrIn (NoErr)"=w302, "IncrSession"=FALSE, "LoadIntf?"=w300, "Interface"=w280) -> ("error out"=w273:errorcluster, "Experiment Path"=w268:path, "Session"=w275:i32, "Interface en sortie"=w304:refnum<class "Interface.lvclass">, "BaseDataPath out"=w267:path)  [unwired: 2 in]
                        n133 = Number To Decimal String(number=w275) -> (decimal integer string=w274:string)  [unwired: 1 in]
                        n134 = call "InitGraphConfig.vi"("Interface en entrée"=w304, "Graph_FA"=w308, "PanRef"=w309, "ListboxRef"=w310, "error in (no error)"=w273, "Graph Event In"=w270, "MainGraphQ In"=w269) -> ("Interface en sortie"=w307:refnum<class "Interface.lvclass">, "error out"=w306:errorcluster)  [unwired: 6 in, 1 out]
                        n135 = Strip Path(path=w268) -> (name=w272:string)  [unwired: 1 out]
                        n136 = call "Initialize.vi"("MainProgQEvent"=w287, "BaseDataPath"=w267, "MainProgQ"=w288, "Experiment Path"=w268, "ErrIn (NoErr)"=w273, "Session"=w282, "SubPanel Refs"=w305, "Experiment In"=w301) -> ("error out"=w293:errorcluster, "PanScanFunc"=w297:string[], "Experiment Out"=w294:refnum<class "Experiment.lvclass">)  [unwired: 1 in]
                        n137 = property on="Interface.lvclass" class="CmdeClasseLV (strict)"(error in=w306, "Value"=w307) -> (error out=w290:errorcluster)  [unwired: 1 in, 1 out]
                        n138 = local write "Experiment Path"(w268) -> ()
                        n139 = Current VI's Menubar() -> (w291:refnum<k9>)
                        n140 = Concatenate Strings("LabScan V1 Session " ("Front Panel Window:Title"), w274, "; " ("string"), w272) -> (w278:string)
                        n141 = call "GetInstrMenuPan.vi"("error in (no error)"=w293, "référence de menu"=w291, "Experiment en entrée"=w294) -> ("error out"=w289:errorcluster, "Experiment en sortie"=w292:refnum<class "Experiment.lvclass">)  [unwired: 7 in]
                        n142 = property on="Scan Function" class="MDér (strict)"(error in=w289, "Strings []"=w297, "Value"=0) -> (error out=w295:errorcluster)  [unwired: 1 in, 1 out]
                        n143 = property class="VI"(error in=w273, "Fenêtre face-avant : titre"=w278) -> ()  [unwired: 1 in, 2 out]
                        n144 = property on="Exper.lvclass" class="CmdeClasseLV (strict)"(error in=w290, "Value"=w292) -> (error out=w311:errorcluster)  [unwired: 1 in, 1 out]
                        n145 = Merge Errors(w311, w295, w285) -> (w296:errorcluster)
                      }
                    }
                  }
                  frame True {
                    n146 = call <vilib>:"Clear Errors.vi"("error in (no error)"=w320) -> ("error out"=w319:errorcluster)  [unwired: 5 in, 1 out]
                  }
                }
              }
              frame "Save Experiment" {
                n147 = local read "Experiment Path"() -> (w328:path)
                n148 = call "SaveInterfSetup.vi"("error in (no error)"=w326, "Experiment Path"=w328, "Interface en entrée"=w327) -> ("error out"=w323:errorcluster, "Cancel Close Out"=w321:bool, "SavePath"=w322:path)  [unwired: 5 in, 1 out]
                n149 = case shown="Faux" w321 {
                  tunnel: w322 -> [w329 _]
                  frame False {
                    n150 = local write "Experiment Path"(w329) -> ()
                  }
                  frame True {
                  }
                }
                n151 = call "SaveExpConfig.vi"("error in (no error)"=w323, "Experiment"=w322, "Experiment.lvclass"=w324) -> ("error out"=w325:errorcluster)  [unwired: 7 in, 1 out]
              }
              frame "LoadNewExpWin" {
                n152 = control-ref of="ce VI"() -> (w353:refnum<vi>)
                n153 = property class="VI"(reference=w353, error in=w350) -> (error out=w351:errorcluster, "Path"=w352:path)  [unwired: 1 out]
                n154 = Open VI Reference(vi path=w352, options=8, error in (no error)=w351) -> (vi reference=w341:refnum<vi>, error out=w336:errorcluster)  [unwired: 3 in]
                n155 = property class="VI"(reference=w341, error in=w336) -> (reference out=w333:refnum<vi>, error out=w335:errorcluster, "Panel"=w340:refnum<vi>)
                n156 = property class="FA"(reference=w340, error in=w335) -> (error out=w334:errorcluster, "Controls[]"=w339:refnum<vi>[])  [unwired: 1 out]
                n157 = To Variant(anything=FALSE) -> (Variant=w331:variant)
                n158 = Index Array(array=w339, index=26) -> (element=w337:refnum<vi>)
                n159 = property class="Cmde"(reference=w337, error in=w334, "Value"=w331) -> (error out=w332:errorcluster)  [unwired: 1 out]
                n160 = invoke class="VI" method="FA.Ouvrir"(reference=w333, error in=w332, "Activate"=TRUE ("Activer ?"), "State"=T4."Standard" ("État")) -> (reference out=w344:refnum<vi>, error out=w345:errorcluster)  [unwired: 1 in, 3 out]
                n161 = invoke class="VI" method="ExécVI"(reference=w344, error in=w345, "Wait until done"=FALSE ("Attendre la fin"), "Auto Dispose Ref"=TRUE ("Supprimer la référence automatiquement")) -> (error out=w346:errorcluster)  [unwired: 1 in, 4 out]
              }
              frame "Config Instruments" {
                n162 = call "SetUpInstruments.vi"("ErrorIn(No Error)"=w357, "Experiment.lvclass"=w356) -> ("sortie d'erreur"=w354:errorcluster, "Experiment.lvclass Out"=w355:refnum<class "Experiment.lvclass">)  [unwired: 8 in]
                n163 = local write "Exper.lvclass"(w355) -> ()
              }
              frame "SetupCalc" {
                n164 = call "SetupCalc.vi"("error in (no error)"=w363, "Experiment.lvclass"=w361, "Interface en entrée"=w360) -> ("error out"=w362:errorcluster, "Experiment.lvclass Out"=w358:refnum<class "Experiment.lvclass">, "Interface en sortie"=w359:refnum<class "Interface.lvclass">)  [unwired: 6 in]
                n165 = local write "Interface.lvclass"(w359) -> ()
                n166 = local write "Exper.lvclass"(w358) -> ()
              }
              frame "CurveEditor" {
                n167 = call "CurveEditor.vi"("error in (no error)"=w369, "Experiment.lvclass"=w367, "Interface en entrée"=w366) -> ("error out"=w368:errorcluster, "Experiment.lvclass Out"=w364:refnum<class "Experiment.lvclass">, "Interface en sortie"=w365:refnum<class "Interface.lvclass">)  [unwired: 6 in]
                n168 = local write "Interface.lvclass"(w365) -> ()
                n169 = local write "Exper.lvclass"(w364) -> ()
              }
              frame "Config Experiment" {
                w380 = 0 ("Function")
                # "&func panel"
                # "need to update scan panel here"
                n170 = control-ref of="ScanFunc"() -> (w370:refnum<vi>)
                n171 = call "SetUpExperiment.vi"("ErrorIn(No Error)"=w386, "ScanTreeIn"=w370, "Exper.lvclass"=w385) -> ("sortie d'erreur"=w383:errorcluster, "Exper.lvclass Out"=w384:refnum<class "Experiment.lvclass">)  [unwired: 7 in]
                n172 = call "UpdateScanPan.vi"("MainProgQEvent"=w373, "MainProgQ"=w374, "error in (no error)"=w383, "Function"=w380, "Experiment en entrée"=w384) -> ("error out"=w381:errorcluster, "PanScanFunc"=w382:string[], "Experiment en sortie"=w376:refnum<class "Experiment.lvclass">)  [unwired: 3 in, 1 out]
                n173 = local write "Exper.lvclass"(w376) -> ()
                n174 = property on="Scan Function" class="MDér (strict)"(error in=w381, "Strings []"=w382, "Value"=w380) -> (error out=w375:errorcluster)  [unwired: 1 in, 1 out]
                n175 = Current VI's Menubar() -> (w377:refnum<k9>)
                n176 = call "GetInstrMenuPan.vi"("error in (no error)"=w375, "référence de menu"=w377, "Experiment en entrée"=w376) -> ("error out"=w371:errorcluster, "Experiment en sortie"=w372:refnum<class "Experiment.lvclass">)  [unwired: 7 in]
                n177 = property class="Interface.lvclass"(reference=w379, "Accessor:Experiment.lvclass"=w372) -> (reference out=w378:refnum<class "Interface.lvclass">)  [unwired: 1 in, 1 out]
                n178 = local write "Interface.lvclass"(w378) -> ()
              }
              frame "Config Interface" {
                n179 = call "SetupInterf.vi"("error in (no error)"=w390, "Experiment.lvclass"=w388, "Interface en entrée"=w387) -> ("error out"=w389:errorcluster, "Interface en sortie"=w391:refnum<class "Interface.lvclass">)  [unwired: 7 in]
                n180 = local write "Interface.lvclass"(w391) -> ()
              }
              frame "SetupGraphConfig" {
                n181 = call "SetupGraphConfig.vi"("Error in"=w397) -> ("error out"=w396:errorcluster, "Canceled"=w392:bool, "GraphConfigOut"=w394:i32)  [unwired: 8 in]
                n182 = case shown="Faux" w392 {
                  tunnel: w396 -> [w402 w403]
                  tunnel: [w401 w403] -> w395
                  tunnel: w394 -> [w400 _]
                  tunnel: w393 -> [w399 _]
                  frame False {
                    n183 = call "ChangeGraphConfig.vi"("error in (no error)"=w402, "NewGraphConfig"=w400, "Interface en entrée"=w399) -> ("error out"=w401:errorcluster, "Interface en sortie"=w398:refnum<class "Interface.lvclass">)  [unwired: 7 in]
                    n184 = local write "Interface.lvclass"(w398) -> ()
                  }
                  frame True {
                  }
                }
              }
              frame "Browse Data" {
                n185 = call <userlib>:"CurrentVIFolder.vi"("error in (no error)"=w414, "Source"=T5."Répertoire du VI actuel", "NomFichier"="Interface Class\\BrowseData.vi") -> ("error out"=w411:errorcluster, "Chemin"=w413:path)  [unwired: 6 in, 1 out]
                n186 = Open VI Reference(type specifier VI Refnum (for type only)=refnum<vi> refnum ("spécificateur de type du refnum de VI (pour type seulement)"), vi path=w413, options=128, error in (no error)=w411) -> (vi reference=w409:refnum<vi>, error out=w407:errorcluster)  [unwired: 2 in]
                n187 = call-by-ref "Démarrer un appel asynchrone"(reference=w409, error in=w407, "MainProgQEvent"=w404, "MainProgQ"=w405, "Interface en entrée"=w408) -> (error out=w406:errorcluster)  [unwired: 7 in, 3 out]
              }
              frame "Paramètres du programme" {
                n188 = call "ParamProg.vi"("ErrorIn(No Error)"=w420, "Interface.lvclass"=w418) -> ("sortie d'erreur"=w419:errorcluster, "Interface.lvclass Out"=w417:refnum<class "Interface.lvclass">)  [unwired: 7 in, 1 out]
                n189 = local write "Interface.lvclass"(w417) -> ()
              }
              frame "Show Class Data" {
                n190 = call "ClassDataEditor.vi"("Experiment.lvclass"=w423, "Interface.lvclass"=w424) -> ("Experiment.lvclass"=w421:refnum<class "Experiment.lvclass">, "Interface.lvclass Out"=w422:refnum<class "Interface.lvclass">)  [unwired: 7 in, 1 out]
                n191 = local write "Interface.lvclass"(w422) -> ()
                n192 = local write "Exper.lvclass"(w421) -> ()
              }
              frame "Data Bindings" {
                n193 = call "DataAssignement.vi"("ErrorIn (NoErr)"=w430, "Experiment.lvclass"=w431) -> ("ErrOut"=w429:errorcluster, "Experiment.lvclassOut"=w427:refnum<class "Experiment.lvclass">)  [unwired: 8 in]
                n194 = call "Get DataBindings.vi"("error in"=w429, "Experiment.lvclass"=w427) -> ("error out"=w428:errorcluster, "Experiment.lvclass out"=w426:refnum<class "Experiment.lvclass">)  [unwired: 8 in]
                n195 = local write "Exper.lvclass"(w426) -> ()
              }
              frame "Quitter" {
                n196 = property on="stop" class="Bool (strict)"(error in=w434, "Valeur (Signalisation)"=TRUE ("Value (Signaling)")) -> (error out=w433:errorcluster)  [unwired: 1 in, 1 out]
              }
              frame "Aide" {
                # "Ouvre le documents d'aide"
                n197 = String To Path(string="") -> (path=w435:path)
                n198 = call-poly <vilib>:"Open URL in Default Browser.vi"("error in (no error)"=w438, "path"=w435) -> ("error out"=w437:errorcluster)  [unwired: 4 in, 1 out]
              }
              frame "À propos" {
                n199 = call "AboutLS1.vi"("error in (no error)"=w440) -> ("error out"=w439:errorcluster)  [unwired: 8 in]
              }
            }
          }
          event "MeasFunc": Double Click {
            n200 = event-data() -> ("CtlRef"=w443:refnum<vi>, "Row"=w444:i32)  [unwired: 1 in]
            n201 = local read "Acq"() -> (w441:bool)
            n202 = case shown="Faux" w441 {
              tunnel: w445 -> [w450 w452]
              tunnel: w444 -> [w449 _]
              tunnel: w443 -> [w448 _]
              tunnel: [w446 w452] -> w442
              frame False {
                n203 = local read "Exper.lvclass"() -> (w451:refnum<class "Experiment.lvclass">)
                n204 = call "SetActiveMeasFunc.vi"("error in (no error)"=w450, "ItemIndex"=w449, "ListRef"=w448, "Experiment en entrée"=w451) -> ("error out"=w446:errorcluster, "Experiment en sortie"=w447:refnum<class "Experiment.lvclass">)  [unwired: 6 in]
                n205 = local write "Exper.lvclass"(w447) -> ()
              }
              frame True {
              }
            }
          }
          event "ScanFunc": Double Click {
            n206 = event-data() -> ("CtlRef"=w456:refnum<vi>, "Tag"=w457:string, "CellPart"=w458:T6)  [unwired: 1 in, 4 out]
            n207 = local read "Acq"() -> (w453:bool)
            n208 = Equal?(x=T6."Text" ("CellPart"), y=w458) -> (x = y?=w460:bool)
            n209 = Equal?(x=T6."Item Symbol" ("CellPart"), y=w458) -> (x = y?=w459:bool)
            n210 = Compound Arithmetic op=OR ("Opérateur arithmétique")(w459, w460) -> (w455:bool)
            n211 = Compound Arithmetic op=AND ("Opérateur arithmétique")(invert w453, w455) -> (w454:bool)
            n212 = case shown="Vrai" w454 {
              tunnel: w464 -> [w465 w471]
              tunnel: [w465 w470] -> w463
              tunnel: w457 -> [_ w467]
              tunnel: w456 -> [_ w469]
              frame False {
              }
              frame True {
                n213 = property class="Arbre (strict)"(reference=w469, "Active Item Tag"=w467) -> (reference out=w466:refnum<vi>, "Indent Level"=w468:i32)  [unwired: 1 in, 1 out]
                n214 = case shown="1" w468 {
                  tunnel: w471 -> [w472 w480]
                  tunnel: [w472 w479] -> w470
                  tunnel: w467 -> [_ w478]
                  tunnel: w466 -> [_ w473]
                  frame 0, Default {
                  }
                  frame 1 {
                    n215 = local read "Scan Function"() -> (w475:u16)
                    n216 = local read "Single Par"() -> (w477:bool)
                    n217 = local read "Exper.lvclass"() -> (w482:refnum<class "Experiment.lvclass">)
                    n218 = call "SetActiveScanFunc.vi"("FuncIndex"=w475, "SingleParMode"=w477, "error in (no error)"=w480, "ScanTag"=w478, "ScanTreeRef"=w473, "Experiment en entrée"=w482) -> ("error out"=w479:errorcluster, "DesactivatedSPM"=w474:bool, "SingleParModeOut"=w476:bool, "Experiment en sortie"=w481:refnum<class "Experiment.lvclass">)  [unwired: 2 in]
                    n219 = case shown="Vrai" w474 {
                      tunnel: w476 -> [_ w483]
                      frame False {
                      }
                      frame True {
                        n220 = local write "Single Par"(w483) -> ()
                      }
                    }
                    n221 = local write "Exper.lvclass"(w481) -> ()
                  }
                }
              }
            }
          }
          event Panel Resize {
            # "go to maximized"
            # "check if we go from maximized to standard"
            # "this check that resize move has ended"
            n222 = event-data() -> ("OldBnds"=w490:T14, "NewBnds"=w489:T14, "Act"=w493:T8, "PrevState"=w492:T7)  [unwired: 1 in]
            n223 = Equal?(x=panelstate."Maximized" ("ÉtatPréc"), y=w492) -> (x = y?=w497:bool)
            n224 = Equal?(x=w493, y=sizeaction."Resized" ("Act")) -> (x = y?=w498:bool)
            n225 = Equal?(x=w493, y=sizeaction."Maximized" ("Act")) -> (x = y?=w485:bool)
            n226 = Equal?(x=w490, y=w489) -> (x = y?=w491:bool)
            n227 = And(x=w497, y=w498) -> (x .and. y?=w484:bool)
            n228 = Compound Arithmetic op=OR(w491, w485, w484) -> (w488:bool)
            n229 = case shown="Vrai" w488 {
              tunnel: w487 -> [w499 w501]
              tunnel: [w499 w500] -> w486
              tunnel: w485 -> [_ _]
              tunnel: w484 -> [_ _]
              frame False {
              }
              frame True {
                n230 = local read "Interface.lvclass"() -> (w502:refnum<class "Interface.lvclass">)
                n231 = call "GraphPanelResize.vi"("error in (no error)"=w501, "Interface en entrée"=w502) -> ("error out"=w500:errorcluster)  [unwired: 8 in, 1 out]
              }
            }
          }
          event "Listbox": Shortcut Menu Selection (User) {
            n232 = event-data() -> ("CtlRef"=w505:refnum<vi>, "ItemTag"=w509:string, "ItemPath"=w506:string)  [unwired: 1 in, 2 out]
            n233 = local read "Interface.lvclass"() -> (w504:refnum<class "Interface.lvclass">)
            n234 = case shown="\"SelAllCrv\"" w509 {
              selector: w509 -> [w510 _ _ _ _ _ _ _]
              tunnel: w508 -> [w515 w591 w601 w609 w642 w655 w666 w674]
              tunnel: [w516 w581 w593 w608 w638 w651 w668 w669] -> w507
              tunnel: w506 -> [_ _ _ _ _ _ _ _]
              tunnel: w505 -> [w514 w583 w592 w610 w643 w656 w667 _]
              tunnel: w504 -> [w513 w587 w596 w607 w640 w653 w663 w672]
              tunnel: [w512 w586 w596 w606 w637 w650 w663 w673] -> w503
              frame Default {
                n235 = Scan From String(format string="Graph %d" ("chaîne de format"), input string=w510, error in=w515) -> (remaining string=w511:string, error out=w518:errorcluster, output 1=w517:i32)  [unwired: 2 in, 1 out]
                n236 = case shown="Pas d'erreur" w518 {
                  selector: w518 -> [w533 w561]
                  tunnel: w517 -> [_ _]
                  tunnel: [w539 w555] -> w516
                  tunnel: w514 -> [w538 w552]
                  tunnel: w513 -> [w527 w558]
                  tunnel: [w537 w557] -> w512
                  tunnel: w511 -> [_ w559]
                  tunnel: w510 -> [w523 _]
                  frame No Error {
                    # "list of all selected curves"
                    # "Handle Graph x click"
                    n237 = property class="LstDér (strict)"(reference=w538, error in=w533) -> (error out=w526:errorcluster, "Value"=w529:i32[])  [unwired: 1 out]
                    n238 = Index Array(array=w529) -> (element=w528:i32)  [unwired: 1 in]
                    n239 = call "GetGraphVIName.vi"("ErrIn (NoErr)"=w526, "Curve Index"=w528, "Interface In"=w527) -> ("error out"=w520:errorcluster, "GraphIndex"=w525:i32, "GraphViNames"=w522:string[], "Interface Out"=w524:refnum<class "Interface.lvclass">)  [unwired: 3 in, 2 out]
                    n240 = Array Size(array=w529) -> (size(s)=w532:i32)
                    n241 = Search 1D Array(1D array=w522, element=w523) -> (index of element=w521:i32)  [unwired: 1 in]
                    n242 = Greater?(x=w532, y=1) -> (0:w530:bool)
                    n243 = case shown="Faux" w530 {
                      tunnel: [w542 w545] -> w534
                      tunnel: w525 -> [w541 _]
                      tunnel: w521 -> [w540 w545]
                      frame False {
                        # "uncheck = no graph(-2)"
                        n244 = Equal?(x=w541, y=w540) -> (x = y?=w543:bool)
                        n245 = Select(t=-2, s=w543, f=w540) -> (s? t:f=w542:i32)
                      }
                      frame True {
                      }
                    }
                    n246 = call "ChangeGraphRefV2.vi"("error in (no error)"=w520, "CurvesIndx"=w529, "NewGraphIndex"=w534, "Interface en entrée"=w524) -> ("error out"=w536:errorcluster, "Interface en sortie"=w535:refnum<class "Interface.lvclass">)  [unwired: 6 in]
                    n247 = for {
                      tunnel: w529 -> [w551] mode=indexing
                      shift-right: [w549] -> w539
                      shift-left: w536 -> [w550]
                      shift-right: [w547] -> w537
                      shift-left: w535 -> [w548]
                      n248 = call "SetCurvVisible.vi"("Force Show"=TRUE ("Force vis"), "error in (no error)"=w550, "CurveIndex"=w551, "Interface en entrée"=w548) -> ("Error out"=w549:errorcluster, "Interface Out"=w547:refnum<class "Interface.lvclass">)  [unwired: 6 in]
                    }
                  }
                  frame Error {
                    # "Selected \"No Graph\"?"
                    n249 = call <vilib>:"Clear Errors.vi"("error in (no error)"=w561) -> ("error out"=w556:errorcluster)  [unwired: 5 in, 1 out]
                    n250 = Match Pattern(string=w559, regular expression="No Graph" ("chaîne de format")) -> (offset past match=w554:i32)  [unwired: 1 in, 3 out]
                    n251 = Greater Or Equal To 0?(x=w554) -> (x >= 0?=w553:bool)
                    n252 = case shown="Vrai" w553 {
                      tunnel: w558 -> [w563 w568]
                      tunnel: [w563 w567] -> w557
                      tunnel: w556 -> [w562 w566]
                      tunnel: [w562 w565] -> w555
                      tunnel: w552 -> [_ w564]
                      frame False {
                      }
                      frame True {
                        n253 = property on="Nœud de propriété" class="LstDér (strict)"(reference=w564, error in=w566) -> (error out=w571:errorcluster, "Value"=w569:i32[])  [unwired: 1 out]
                        n254 = call "ChangeGraphRefV2.vi"("error in (no error)"=w571, "CurvesIndx"=w569, "NewGraphIndex"=-2, "Interface en entrée"=w568) -> ("error out"=w573:errorcluster, "Interface en sortie"=w572:refnum<class "Interface.lvclass">)  [unwired: 6 in]
                        n255 = for {
                          tunnel: w569 -> [w579] mode=indexing
                          shift-right: [w577] -> w565
                          shift-left: w573 -> [w578]
                          shift-right: [w575] -> w567
                          shift-left: w572 -> [w576]
                          n256 = call "SetCurvVisible.vi"("Force Show"=FALSE ("Force vis"), "error in (no error)"=w578, "CurveIndex"=w579, "Interface en entrée"=w576) -> ("Error out"=w577:errorcluster, "Interface Out"=w575:refnum<class "Interface.lvclass">)  [unwired: 6 in]
                        }
                      }
                    }
                  }
                }
              }
              frame "SelScanCrv" {
                n257 = property on="Listbox" class="LstDér (strict)"(error in=w591) -> (error out=w588:errorcluster, "Value"=w590:i32[])  [unwired: 1 in, 1 out]
                n258 = Index Array(array=w590) -> (element=w589:i32)  [unwired: 1 in]
                n259 = call "GetScanCrvInd.vi"("error in (no error)"=w588, "Curve Ind"=w589, "Interface.lvclass"=w587) -> ("error out"=w585:errorcluster, "Curves Index"=w584:i32[], "Interface.lvclass Out"=w586:refnum<class "Interface.lvclass">)  [unwired: 6 in]
                n260 = property on="Listbox" class="LstDér (strict)"(error in=w585, "Value"=w584) -> (error out=w582:errorcluster)  [unwired: 1 in, 1 out]
                n261 = property class="LstDér (strict)"(reference=w583, error in=w582, "Key Focus"=TRUE ("Focus clavier")) -> (error out=w581:errorcluster)  [unwired: 1 out]
              }
              frame "SelAllCrv" {
                n262 = property on="Listbox" class="LstDér (strict)"(error in=w601) -> (error out=w597:errorcluster, "Item Names"=w600:string[])  [unwired: 1 in, 1 out]
                n263 = Array Size(array=w600) -> (size(s)=w599:i32)
                n264 = for {
                  N: w599 -> [_]
                  tunnel: [w602] -> w598 mode=indexing
                  i -> [w602]
                }
                n265 = property on="Listbox" class="LstDér (strict)"(error in=w597, "Value"=w598) -> (error out=w594:errorcluster)  [unwired: 1 in, 1 out]
                n266 = property class="LstDér (strict)"(reference=w592, error in=w594, "Key Focus"=TRUE ("Focus clavier")) -> (error out=w593:errorcluster)  [unwired: 1 out]
              }
              frame "OpenData" {
                n267 = property class="LstDér (strict)"(reference=w610, error in=w609) -> (error out=w603:errorcluster, "Value"=w605:i32[])  [unwired: 1 out]
                n268 = for {
                  shift-right: [w622] -> w606
                  shift-left: w607 -> [w623]
                  tunnel: w605 -> [w621] mode=indexing
                  shift-right: [w624] -> w608
                  shift-left: w603 -> [w620]
                  shift-right: [w617] -> _
                  shift-left: path[] [] -> [w615]
                  n269 = call "GetCurvesParams.vi"("error in (no error)"=w620, "CurvIndex"=w621, "Interface en entrée"=w623) -> ("error out"=w619:errorcluster, "CurvePar Out"=w618:T16, "Interface en sortie"=w622:refnum<class "Interface.lvclass">)  [unwired: 6 in]
                  n270 = Unbundle By Name(w618) -> ("File Path"=w613:path)
                  n271 = Search 1D Array(1D array=w615, element=w613) -> (index of element=w616:i32)  [unwired: 1 in]
                  n272 = Greater Or Equal To 0?(x=w616) -> (x >= 0?=w614:bool)
                  n273 = Empty String/Path?(string/path=w613) -> (empty?=w612:bool)
                  n274 = Or(x=w612, y=w614) -> (x .or. y?=w611:bool)
                  n275 = case shown="Faux" w611 {
                    tunnel: [w634 w636] -> w624
                    tunnel: w619 -> [w633 w636]
                    tunnel: [w627 w635] -> w617
                    tunnel: w613 -> [w626 _]
                    tunnel: w615 -> [w625 w635]
                    frame False {
                      n276 = Path To String(path=w626) -> (string=w629:string)
                      n277 = Build Array (concatenate)(w625, w626) -> (w627:path[])
                      n278 = Concatenate Strings("notepad" ("command line"), " " ("string"), w629) -> (w628:string)
                      n279 = call <vilib>:"System Exec.vi"("wait until completion? (T)"=FALSE, "error in (no error)"=w633, "command line"=w628) -> ("error out"=w634:errorcluster)  [unwired: 5 in, 3 out]
                    }
                    frame True {
                    }
                  }
                }
              }
              frame "ShowCrv" {
                n280 = property class="LstDér (strict)"(reference=w643, error in=w642) -> (error out=w639:errorcluster, "Value"=w641:i32[])  [unwired: 1 out]
                n281 = for {
                  tunnel: w641 -> [w649] mode=indexing
                  shift-right: [w646] -> w637
                  shift-left: w640 -> [w647]
                  shift-right: [w644] -> w638
                  shift-left: w639 -> [w645]
                  n282 = call "SetCurvVisible.vi"("Force Show"=TRUE ("Force vis"), "error in (no error)"=w645, "CurveIndex"=w649, "Interface en entrée"=w647) -> ("Error out"=w644:errorcluster, "Interface Out"=w646:refnum<class "Interface.lvclass">)  [unwired: 6 in]
                }
              }
              frame "HideCrv" {
                n283 = property class="LstDér (strict)"(reference=w656, error in=w655) -> (error out=w652:errorcluster, "Value"=w654:i32[])  [unwired: 1 out]
                n284 = for {
                  tunnel: w654 -> [w662] mode=indexing
                  shift-right: [w660] -> w650
                  shift-left: w653 -> [w661]
                  shift-right: [w658] -> w651
                  shift-left: w652 -> [w659]
                  n285 = call "SetCurvVisible.vi"("Force Hide"=TRUE, "error in (no error)"=w659, "CurveIndex"=w662, "Interface en entrée"=w661) -> ("Error out"=w658:errorcluster, "Interface Out"=w660:refnum<class "Interface.lvclass">)  [unwired: 6 in]
                }
              }
              frame "ExPython" {
                n286 = property class="LstDér (strict)"(reference=w667, error in=w666) -> (error out=w665:errorcluster, "Value"=w664:i32[])  [unwired: 1 out]
                n287 = call "CurveExport.vi"("error in (no error)"=w665, "Curves"=w664, "Interface en entrée"=w663) -> ("error out"=w668:errorcluster)  [unwired: 8 in]
              }
              frame "OpenNewGraph" {
                n288 = property on="Listbox" class="LstDér (strict)"(error in=w674) -> (error out=w670:errorcluster, "Value"=w671:i32[])  [unwired: 1 in, 1 out]
                n289 = call "NewGrphWindow.vi"("error in (no error)"=w670, "CurvesIndx"=w671, "Interface en entrée"=w672) -> ("error out"=w669:errorcluster, "Interface en sortie"=w673:refnum<class "Interface.lvclass">)  [unwired: 7 in]
              }
            }
            n290 = local write "Interface.lvclass"(w503) -> ()
          }
          event User Event {
            n291 = event-data() -> ("UsrEvtRef"=w676:refnum<user-event>, "queue out"=w679:refnum<queue>)  [unwired: 1 in]
            n292 = local read "Exper.lvclass"() -> (w682:refnum<class "Experiment.lvclass">)
            n293 = local read "Interface.lvclass"() -> (w678:refnum<class "Interface.lvclass">)
            n294 = Dequeue Element(queue=w679, error in (no error)=w681) -> (element=w687:cluster{"Message":string, "Data":variant, i32}, error out=w680:errorcluster)  [unwired: 1 in, 2 out]
            n295 = Unbundle(w687) -> ("Message"=w686:string, "Data"=w685:variant)  [unwired: 1 out]
            n296 = case shown="\"ArrDevAcq\"" w686 {
              selector: w686 -> [w689 _ _ _ _ _ _ _]
              tunnel: w685 -> [w696 w702 w708 _ _ w728 w754 w772]
              tunnel: w680 -> [w697 w703 w709 w711 w714 w727 w755 w770]
              tunnel: [w692 w700 w704 w711 w714 w729 w756 w762] -> w684
              tunnel: [w694 w699 w707 w712 w715 w739 w748 w766] -> w683
              tunnel: w682 -> [w695 w699 w707 w712 w715 w741 w748 w783]
              tunnel: w679 -> [_ _ _ _ _ w733 _ _]
              tunnel: w678 -> [w688 w701 _ w710 w713 w737 w750 w782]
              tunnel: [w688 w701 w705 w710 w713 w736 w749 w761] -> w677
              tunnel: w676 -> [_ _ _ _ _ w732 _ _]
              tunnel: w675 -> [_ _ _ _ _ _ _ _]
              frame "", Default {
                n297 = Variant To Data(error in=w697, type=refnum<class "BaseDevice.lvclass"> refnum ("BaseDevice.lvclass"), Variant=w696) -> (data=w690:refnum<class "BaseDevice.lvclass">, error out=w693:errorcluster)
                n298 = call "UpdateInstrClass.vi"("error in (no error)"=w693, "Message"=w689, "BaseDevice Class"=w690, "Experiment en entrée"=w695) -> ("error out"=w692:errorcluster, "Experiment en sortie"=w694:refnum<class "Experiment.lvclass">)  [unwired: 6 in]
              }
              frame "SetMeasFunc" {
                n299 = Variant To Data(error in=w703, type=string[] [], Variant=w702) -> (error out=w700:errorcluster)  [unwired: 1 out]
              }
              frame "UpdateItf" {
                n300 = Variant To Data(error in=w709, type=refnum<class "Interface.lvclass"> refnum ("Interface.lvclass"), Variant=w708) -> (data=w705:refnum<class "Interface.lvclass">, error out=w704:errorcluster)
              }
              frame "UpdateScanTime" {
              }
              frame "RequestUpdate" {
              }
              frame "ArrayDevAcqSetup" {
                n301 = Variant To Data(error in=w727, type=cluster{string, bool} {"", TRUE}, Variant=w728) -> (data=w726:cluster{string, bool}, error out=w725:errorcluster)
                n302 = Unbundle(w726) -> (w723:string, w718:bool)
                n303 = local read "DescKword"() -> (w721:string)
                n304 = call "SetArrayDevParams.vi"("Interface.lvclass"=w737, "DescKword"=w721, "Save"=w718, "Experiment.lvclass"=w741, "error in"=w725, "ArrayFuncName"=w723) -> ("DataFileRef"=w738:refnum<file>, "Interf.lvclass Out"=w747:refnum<class "Interface.lvclass">, "DataFileName"=w720:path, "DevId"=w717:i32, "Exp.lvclass Out"=w739:refnum<class "Experiment.lvclass">, "Scan list"=w740:string[], "error out"=w746:errorcluster)  [unwired: 3 in]
                n305 = local write "ScanList"(w740) -> ()
                n306 = local write "DataFileRef"(w738) -> ()
                n307 = local write "path"(w720) -> ()
                n308 = call "GraphSetup.vi"("error in"=w746, "AllowDef"=TRUE, "DataFileName"=w720, "InterfaceIn"=w747) -> ("error out"=w743:errorcluster, "InterfaceOut"=w745:refnum<class "Interface.lvclass">)  [unwired: 6 in]
                n309 = Bundle(w718, "DevId"=w717) -> (w716:cluster{bool, "DevId":i32})  [unwired: 1 in]
                n310 = call "2DGraphSetup.vi"("error in (no error)"=w743, "Interface en entrée"=w745) -> ("error out"=w742:errorcluster, "Interface en sortie"=w744:refnum<class "Interface.lvclass">)  [unwired: 8 in]
                n311 = Bundle By Name(cluster=T9 {"Message"="ArrDevAcq", "Data"=variant, "Code"=0} ("élément"), "Data"=w716) -> (w722:T9)
                n312 = call "AddtoCurveList.vi"("error in (no error)"=w742, "Interface en entrée"=w744) -> ("error out"=w735:errorcluster, "Interface en sortie"=w736:refnum<class "Interface.lvclass">)  [unwired: 8 in]
                n313 = Enqueue Element(queue=w733, element=w722, error in (no error)=w735) -> (queue out=w731:refnum<queue>, error out=w730:errorcluster)  [unwired: 1 in, 1 out]
                n314 = Generate User Event(user event=w732, event data cluster=w731, error in=w730) -> (error out=w729:errorcluster)  [unwired: 1 in, 1 out]
              }
              frame "ClearGraph" {
                n315 = Variant To Data(error in=w755, type=0, Variant=w754) -> (data=w751:i32, error out=w753:errorcluster)
                n316 = call "ClearGraphData.vi"("error in (no error)"=w753, "GraphNumber"=w751, "Interface en entrée"=w750) -> ("error out"=w756:errorcluster, "Interface en sortie"=w749:refnum<class "Interface.lvclass">)  [unwired: 6 in, 1 out]
              }
              frame "ArrDevAcq" {
                (unwired) TRUE
                w780 = 0 ("IndicePoint")
                # "refresh graphs"
                # "write calc q"
                # "write data q"
                # "acquire data"
                n317 = Variant To Data(error in=w770, type=cluster{bool, "DevId":i32} {FALSE, "DevId"=0} ("cluster de sortie"), Variant=w772) -> (data=w771:cluster{bool, "DevId":i32}, error out=w769:errorcluster)
                n318 = Unbundle(w771) -> (w759:bool, "DevId"=w758:i32)
                n319 = call "Measure.vi"("DevId"=w758, "error in"=w769, "Scan"=FALSE, "IndicePoint"=w780, "Experiment.lvclass In"=w783) -> ("error out"=w781:errorcluster, "ArrDevDat"=w773:T17[], "Experiment.lvclass Out"=w767:refnum<class "Experiment.lvclass">, "SaveArrVarPar"=w768:bool[], "MeasTimes"=w757:u32[])  [unwired: 1 in, 1 out]
                n320 = call "WriteArrDataSingleRun.vi"("SaveArrVarPar"=w768, "IndPoint"=w780, "error in (no error)"=w781, "ArrDevDat"=w773, "Save"=w759, "Interface en entrée"=w782) -> ("error out"=w778:errorcluster, "Interface en sortie"=w779:refnum<class "Interface.lvclass">)  [unwired: 2 in, 2 out]
                n321 = local write "MeasTimes"(w757) -> ()
                n322 = call "RefreshGraphArr.vi"("error in (no error)"=w778, "Interface en entrée"=w779) -> ("error out"=w774:errorcluster, "Interface en sortie"=w775:refnum<class "Interface.lvclass">)  [unwired: 8 in]
                n323 = call "IncrCurveInd.vi"("error in (no error)"=w774, "Interface en entrée"=w775) -> ("error out"=w777:errorcluster, "Interface en sortie"=w776:refnum<class "Interface.lvclass">)  [unwired: 8 in]
                n324 = call "SaveDataQRef.vi"("error in (no error)"=w777, "Interface.lvclass"=w776) -> ("error out"=w765:errorcluster, "Interface.lvclass Out"=w761:refnum<class "Interface.lvclass">)  [unwired: 8 in]
                n325 = call "EndScan.vi"("error in (no error)"=w765, "AcqComp"=TRUE, "Experiment en entrée"=w767) -> ("error out"=w762:errorcluster, "Experiment en sortie"=w766:refnum<class "Experiment.lvclass">)  [unwired: 6 in, 1 out]
              }
            }
            n326 = local write "Interface.lvclass"(w677) -> ()
            n327 = local write "Exper.lvclass"(w683) -> ()
          }
          event "refresh test": Value Change {
            n328 = event-data() -> ("NewVal"=w784:bool)  [unwired: 1 in, 5 out]
            n329 = control-ref of="FA_G1"() -> (w785:refnum<vi>)
            n330 = property class="FAsec"(reference=w785, "SyncDisp"=w784) -> ()  [unwired: 1 in, 2 out]
          }
          event "Listbox": Shortcut Menu Activation? {
            n331 = event-data() -> ("MenuRef"=w802:refnum<k9>, "CtlRef"=w801:refnum<vi>)  [unwired: 1 in]
            n332 = property class="LstDér (strict)"(reference=w801, error in=w800) -> (error out=w799:errorcluster, "Value"=w798:i32[])  [unwired: 1 out]
            n333 = local read "Interface.lvclass"() -> (w787:refnum<class "Interface.lvclass">)
            n334 = Array Size(array=w798) -> (size(s)=w792:i32)
            n335 = Greater Than 0?(x=w792) -> (x > 0?=w791:bool)
            n336 = Equal?(x=w792, y=1) -> (x = y?=w797:bool)
            n337 = Select(t=T10."Many Items Sel", s=w791, f=T10."No Item Sel") -> (s? t:f=w788:T10)
            n338 = Select(t=T10."One Item Sel", s=w797, f=w788) -> (s? t:f=w794:T10)
            n339 = case shown="\"No Item Sel\", Par défaut" w794 {
              tunnel: w802 -> [_ w826 w845]
              tunnel: w799 -> [w805 w822 w844]
              tunnel: w798 -> [_ w821 _]
              tunnel: [w805 w818 w843] -> w795
              tunnel: w787 -> [w804 w811 w842]
              tunnel: [w804 w810 w834] -> w786
              frame "No Item Sel", Default {
              }
              frame "One Item Sel" {
                w807 = string[] ["Select All Curves", "Select Scan Curves", "Hide Curve", "Show Curve", "Show in New Graph Window", "Open Curve's Data", "Export to Python", "APP_SEPARATOR", "Show On Graph:"] ("tableau ajouté")
                # "select the Graph x elements"
                # "coche l'élément"
                n340 = Index Array(array=w821) -> (element=w816:i32)  [unwired: 1 in]
                n341 = call "GetGraphVIName.vi"("ErrIn (NoErr)"=w822, "Curve Index"=w816, "Interface In"=w811) -> ("error out"=w825:errorcluster, "GraphIndex"=w808:i32, "GraphViNames"=w809:string[], "Interface Out"=w810:refnum<class "Interface.lvclass">)  [unwired: 3 in, 2 out]
                n342 = Array Size(array=w807) -> (size(s)=w806:i32)
                n343 = Build Array (concatenate)(w807, w809) -> (w819:string[])
                n344 = Build Array (concatenate)(string[] ["SelAllCrv", "SelScanCrv", "HideCrv", "ShowCrv", "OpenNewGraph", "OpenData", "ExPython", "APP_SEPARATOR", "ShowOnGraph"] ("tableau ajouté"), w809) -> (w812:string[])
                n345 = Insert Menu Items(4:"100" ("élément suivant"), 6:w825, 7:w812, 8:w819, 9:w826) -> (0:w820:errorcluster, 1:w817:string[], 3:w824:refnum<k9>)  [unwired: 1 in]
                n346 = Delete From Array(array=w817, length=w806, index=0 ("indice")) -> (array with subset deleted=w814:string[])  [unwired: 1 out]
                n347 = for {
                  tunnel: w824 -> [w833]
                  tunnel: w814 -> [w832] mode=indexing
                  tunnel: w808 -> [w830]
                  shift-right: [w827] -> w818
                  shift-left: w820 -> [w828]
                  i -> [w831]
                  n348 = Equal?(x=w830, y=w831) -> (x = y?=w829:bool)
                  n349 = Set Menu Item Info(6:w829, 7:w832, 8:w828, 11:w833) -> (0:w827:errorcluster)  [unwired: 3 in, 1 out]
                }
              }
              frame "Many Items Sel" {
                n350 = call "GetGraphVIName.vi"("Interface In"=w842) -> ("GraphViNames"=w839:string[], "Interface Out"=w834:refnum<class "Interface.lvclass">)  [unwired: 5 in, 4 out]
                n351 = Build Array (concatenate)(w839, "No Graph" ("Front Panel.Title")) -> (w838:string[])
                n352 = Build Array (concatenate)(string[] ["OpenNewGraph", "HideCrv", "ShowCrv", "ExPython", "APP_SEPARATOR", "ShowOnGraph"] ("tableau ajouté"), w838) -> (w835:string[])
                n353 = Build Array (concatenate)(string[] ["Show in New Graph Window", "Hide Curves", "Show Curves", "Export to Python", "APP_SEPARATOR", "Show On Graph:"] ("tableau ajouté"), w838) -> (w836:string[])
                n354 = Insert Menu Items(4:"100" ("élément suivant"), 6:w844, 7:w835, 8:w836, 9:w845) -> (0:w843:errorcluster)  [unwired: 1 in, 2 out]
              }
            }
            n355 = local write "Interface.lvclass"(w786) -> ()
            n356 = event-data("Discard?"=FALSE ("Rejeter ?")) -> ()  [unwired: 1 in, 1 out]
          }
          event "Acq": Mouse Down? {
            # "Bouton balayage"
            n357 = event-data() -> ()  [unwired: 1 in, 1 out]
            n358 = local read "sem1"() -> (w851:T1)
            n359 = case shown="Faux" "Pause" {
              tunnel: [w862 TRUE] -> w847
              tunnel: w848 -> [w855 w952]
              tunnel: w851 -> [w861 w951]
              tunnel: [w860 w948] -> w849
              frame False {
                n360 = call <vilib>:"Acquire Semaphore.vi"("error in (no error)"=w855, "semaphore"=w861) -> ("error out"=w858:errorcluster, "semaphore out"=w859:T1)  [unwired: 3 in, 1 out]
                n361 = local read "Scan Function"() -> (w853:u16)
                n362 = local read "Single Par"() -> (w852:bool)
                n363 = flat-sequence {
                  tunnel: [w865] -> w857
                  tunnel: w859 -> [w864]
                  tunnel: [w864] -> w856
                  tunnel: w858 -> [w863]
                  tunnel: [w863] -> w854
                  frame #0 {
                    n364 = local read "Acq"() -> (w865:bool)
                  }
                }
                n365 = case shown="Faux" w857 {
                  tunnel: [w877 w926] -> w862
                  tunnel: w856 -> [w875 w928]
                  tunnel: [w876 w927] -> w860
                  tunnel: w854 -> [w874 w918]
                  tunnel: w853 -> [w868 _]
                  tunnel: w852 -> [w867 _]
                  frame False {
                    # "On demande le démarrage de l'acquisition"
                    n366 = local read "Exper.lvclass"() -> (w871:refnum<class "Experiment.lvclass">)
                    n367 = To Long Integer(number=w868) -> (32bit integer=w866:i32)
                    n368 = call <vilib>:"Release Semaphore.vi"("error in (no error)"=w874, "semaphore"=w875) -> ("error out"=w872:errorcluster)  [unwired: 4 in, 1 out]
                    n369 = call "SetPosTables.vi"("Error in (no err)"=w872, "ScanFunc"=w866, "SinglePar"=w867, "Experiment In"=w871) -> ("error out"=w873:errorcluster, "NbPos"=w869:i32, "Experiment Out"=w870:refnum<class "Experiment.lvclass">)  [unwired: 5 in]
                    n370 = local write "nb pos"(w869) -> ()
                    n371 = case shown="Pas d'erreur" w873 {
                      selector: w873 -> [w887 w915]
                      tunnel: [w897 TRUE ("T button?")] -> w877
                      tunnel: [w898 w911] -> w876
                      tunnel: w870 -> [w905 _]
                      tunnel: w866 -> [w894 _]
                      tunnel: w867 -> [w893 _]
                      frame No Error {
                        # "Bouton à désactivé>"
                        n372 = local read "DescKword"() -> (w892:string)
                        n373 = call "SetScanParams.vi"("ScanFunc"=w894, "DescKword"=w892, "error in"=w887, "Experiment.lvclass"=w905, "SinglePar"=w893, "Interface.lvclass"="Interface.lvclass") -> ("error out"=w878:errorcluster, "Experiment.lvclass Out"=w882:refnum<class "Experiment.lvclass">, "DataFileName"=w879:path, "Interface.lvclass Out"=w906:refnum<class "Interface.lvclass">, "Scan list"=→"ScanList":string[], "DataFileRef"=w908:refnum<file>)
                        n374 = control-ref of="Discard"() -> (w884:refnum<vi>)
                        n375 = control-ref of="stop"() -> (w880:refnum<vi>)
                        n376 = call "GraphSetup.vi"("error in"=w878, "DataFileName"=w879, "InterfaceIn"=w906) -> ("error out"=w900:errorcluster, "InterfaceOut"=w902:refnum<class "Interface.lvclass">)  [unwired: 7 in]
                        n377 = local write "DataFileRef"(w908) -> ()
                        n378 = local write "path"(w879) -> ()
                        n379 = call "2DGraphSetup.vi"("error in (no error)"=w900, "Interface en entrée"=w902) -> ("error out"=w899:errorcluster, "Interface en sortie"=w901:refnum<class "Interface.lvclass">)  [unwired: 8 in]
                        n380 = call "AddtoCurveList.vi"("error in (no error)"=w899, "Interface en entrée"=w901) -> ("error out"=w891:errorcluster, "Interface en sortie"=w889:refnum<class "Interface.lvclass">)  [unwired: 8 in]
                        n381 = Build Array(w884, w880) -> (w881:refnum<vi>[])
                        n382 = Current VI's Menubar() -> (w910:refnum<k9>)
                        n383 = call <userlib>:"GestionMenuGen.vi"("error in"=w878, "ToDisableItems"=string[] ["Save Experiment", "Quitter LabScan", "Config Instruments", "Config Experiment", "Config Interface", "SetupGraphConfig", "SetupCalc", "Paramètres du programme", "Data Bindings"], "référence de menu"=w910) -> ("error Out"=w895:errorcluster)  [unwired: 8 in]
                        n384 = call "SaveDataQRef.vi"("error in (no error)"=w891, "Interface.lvclass"=w889) -> ("error out"=w890:errorcluster, "Interface.lvclass Out"=w888:refnum<class "Interface.lvclass">)  [unwired: 8 in]
                        n385 = call-poly <userlib>:"SetCtrlPropGenPol.vi"("Error in"=w878, "Énum"=T2."DisAndGrayed", "Controls"=w881) -> ("Error out"=w886:errorcluster)  [unwired: 3 in, 1 out]
                        n386 = local write "Interface.lvclass"(w888) -> ()
                        n387 = call "SignalAcqStatus.vi"("error in (no error)"=w890, "Booléen"=TRUE, "Experiment en entrée"=w882) -> ("error out"=w896:errorcluster, "Experiment en sortie"=w904:refnum<class "Experiment.lvclass">)  [unwired: 7 in]
                        n388 = Merge Errors(w896, w895, w886) -> (w898:errorcluster)
                        n389 = local write "Exper.lvclass"(w904) -> ()
                        n390 = Unbundle By Name(w898) -> ("status"=w897:bool)
                      }
                      frame Error {
                        w912 = 1 items=["pas d'exception", "annuler l'erreur sur correspondance", "définir l'erreur sur correspondance"] ("[exception action] (none:0)")
                        w914 = T15 0 items=["pas de dialogue", "Message OK", "Message continuer ou arrêter", "Message OK + mises en garde", "Arrêter/Continuer + mises en garde"] ("type of dialog (OK msg:1)")
                        # "Paramètres de scan invalides"
                        n391 = call <vilib>:"General Error Handler.vi"("type of dialog (OK msg:1)"=w914, "error in (no error)"=w915, "[exception action] (none:0)"=w912, "[exception code]"=0) -> ("error out"=w911:errorcluster)  [unwired: 7 in, 4 out]
                      }
                    }
                  }
                  frame True {
                    # "on demande l'arrêt"
                    # "Ici, durant l'affichage de la boîte de dialogue,la boucle d'acquisition est en attente, dû au fait que la sémaphore est vérouillé."
                    # "on demande l'arrêt de l'aquisition"
                    n392 = local read "Exper.lvclass"() -> (w917:refnum<class "Experiment.lvclass">)
                    n393 = call <vilib>:"Three Button Dialog.vi"("Allow user to close window? (TRUE)"=FALSE, "Window Title (\"\")"="Arrêt du Balayage" ("Window Title (\"\")"), "Right Button Text (\"Cancel\")"="Pause" ("F button name (\"Cancel\")"), "Center Button Text (\"No\")"="Continuer" ("F button name (\"Cancel\")"), "Left Button Text (\"Yes\")"="Arrêter" ("T button name (\"OK\")"), "message"="L'acquisition est en cours d'arrêt\nPour terminer définitivement l'acquisition, appuyer sur Arrêter\nPour reprendre l'acquisition maintenant, appuyer sur Continuer\nPour faire une pause et reprendre ultérieurement, appuyer sur  Pause et réappuyer sur \"Balayage\" pour reprendre") -> ("Which Button?"=w920:T18)  [unwired: 5 in]
                    n394 = case shown="\"Left Button\"" w920 {
                      tunnel: w928 -> [w935 w944 _]
                      tunnel: w918 -> [w934 w943 w947]
                      tunnel: [w931 w942 w946] -> w927
                      tunnel: [TRUE TRUE w945] -> w926
                      tunnel: w917 -> [w930 _ _]
                      frame "Left Button" {
                        # "on désire arrêter"
                        n395 = flat-sequence {
                          tunnel: w935 -> [w940]
                          tunnel: [w940] -> w936
                          tunnel: w934 -> [w939]
                          tunnel: [w939] -> w937
                          frame #0 {
                            n396 = local write "AcqStop"(TRUE) -> ()
                          }
                        }
                        n397 = call <vilib>:"Release Semaphore.vi"("error in (no error)"=w937, "semaphore"=w936) -> ("error out"=w932:errorcluster)  [unwired: 4 in, 1 out]
                        n398 = call "SignalAcqDev.vi"("error in (no error)"=w932, "Message"=cluster{"Message":string, "Data":variant, i32} {"Message"="ForceStop", "Data"=variant, 0}, "Experiment en entrée"=w930) -> ("error out"=w931:errorcluster)  [unwired: 7 in, 1 out]
                      }
                      frame "Center Button", Default {
                        # "on désire continuer"
                        n399 = call <vilib>:"Release Semaphore.vi"("error in (no error)"=w943, "semaphore"=w944) -> ("error out"=w942:errorcluster)  [unwired: 4 in, 1 out]
                      }
                      frame "Right Button" {
                        w945 = TRUE ("Blinking")
                        # "on fait une pause"
                        n400 = property on="Acq" class="Bool (strict)"(error in=w947, "Clignotant"=w945) -> (error out=w946:errorcluster)  [unwired: 1 in, 1 out]
                        n401 = local write "Pause"(w945) -> ()
                      }
                    }
                  }
                }
              }
              frame True {
                w949 = FALSE ("Blinking")
                # "on demande le redémarrage (fin de pause)"
                n402 = property on="Acq" class="Bool (strict)"(error in=w952, "Clignotant"=w949) -> (error out=w953:errorcluster)  [unwired: 1 in, 1 out]
                n403 = local write "Pause"(w949) -> ()
                n404 = call <vilib>:"Release Semaphore.vi"("error in (no error)"=w953, "semaphore"=w951) -> ("error out"=w948:errorcluster)  [unwired: 4 in, 1 out]
              }
            }
            n405 = event-data("Discard?"=w847) -> ()  [unwired: 4 in, 1 out]
          }
          event "Discard": Value Change {
            n406 = event-data() -> ("NewVal"=w957:bool)  [unwired: 1 in, 5 out]
            n407 = case shown="Vrai" w957 {
              tunnel: w956 -> [w958 w963]
              tunnel: [w958 w962] -> w955
              tunnel: [_ FALSE] -> w954
              frame False {
              }
              frame True {
                n408 = Two Button Dialog(message="This will remove the last scan data from the program and erase it's data file from disk. Proceed?") -> (T button?=w960:bool)  [unwired: 2 in]
                n409 = case shown="Vrai" w960 {
                  tunnel: w963 -> [w964 w966]
                  tunnel: [w964 w965] -> w962
                  frame False {
                  }
                  frame True {
                    n410 = local read "Interface.lvclass"() -> (w968:refnum<class "Interface.lvclass">)
                    n411 = call "DiscardData.vi"("error in (no err)"=w966, "Interface In"=w968) -> ("error out"=w965:errorcluster, "Interface Out"=w967:refnum<class "Interface.lvclass">)  [unwired: 8 in]
                    n412 = local write "Interface.lvclass"(w967) -> ()
                  }
                }
              }
            }
            n413 = local write "Discard"(w954) -> ()
          }
          event User Event {
            n414 = event-data() -> ("queue out"=w977:refnum<queue>)  [unwired: 1 in, 4 out]
            n415 = Dequeue Element(queue=w977, error in (no error)=w976) -> (element=w975:cluster{"Message":string, "Data":variant, i32}, error out=w972:errorcluster)  [unwired: 1 in, 2 out]
            n416 = local read "Interface.lvclass"() -> (w969:refnum<class "Interface.lvclass">)
            n417 = Unbundle By Name(w975) -> ("Data"=w973:variant, "Message"=w974:string)
            n418 = case shown="\"Goto2DGraphPos\"" w974 {
              tunnel: w973 -> [_ w986 w1002 w1010 w1016 w1044 w1051]
              tunnel: w972 -> [w979 w983 w1001 w1009 w1015 w1043 w1050]
              tunnel: [w979 w982 w1000 w1005 w1012 w1040 w1048] -> w971
              tunnel: [w978 w981 w999 w1003 w1013 w1039 w1046] -> w970
              tunnel: w969 -> [w978 w980 w998 w1004 w1014 w1033 w1047]
              frame Default {
              }
              frame "ClearGraph" {
                n419 = Two Button Dialog(message="This will erase all curves from data list ") -> (T button?=w984:bool)  [unwired: 2 in]
                n420 = case shown="Vrai" w984 {
                  tunnel: w986 -> [_ w995]
                  tunnel: w983 -> [w988 w992]
                  tunnel: [w988 w991] -> w982
                  tunnel: [w987 w990] -> w981
                  tunnel: w980 -> [w987 w989]
                  frame False {
                  }
                  frame True {
                    n421 = Variant To Data(type=0, Variant=w995) -> (data=w993:i32)  [unwired: 1 in, 1 out]
                    n422 = call "ClearGraphData.vi"("error in (no error)"=w992, "GraphNumber"=w993, "Interface en entrée"=w989) -> ("error out"=w991:errorcluster, "Interface en sortie"=w990:refnum<class "Interface.lvclass">)  [unwired: 6 in, 1 out]
                  }
                }
              }
              frame "ClearGraphInt" {
                n423 = Variant To Data(type=0, Variant=w1002) -> (data=w996:i32)  [unwired: 1 in, 1 out]
                n424 = call "ClearGraphData.vi"("error in (no error)"=w1001, "GraphNumber"=w996, "Interface en entrée"=w998) -> ("error out"=w1000:errorcluster, "Interface en sortie"=w999:refnum<class "Interface.lvclass">)  [unwired: 6 in, 1 out]
              }
              frame "PlotChange" {
                # "One of the plots attribute's have been changed through the graphical interface. Make interface class reflect these changes"
                n425 = Variant To Data(error in=w1009, type=T11 {"PlotIdx"=0, "PlotAttrib"={"Color"=0, "PointStyle"=0, "LineStyle"=0, "Interp"=0, "LineWidth"=0, "BarPlotStyle"=0, "FillTo"=0, "XScaleIdx"=0, "YScaleIdx"=0, "Anti-Aliased"=FALSE, "LabelFormat"=0, "TransitionType"=0, "TransitionLocation"=0, "DigitalLineStyle"=0}, "GraphId"=0, "Crv Visible"=FALSE} ("PlotChange"), Variant=w1010) -> (data=w1007:T11, error out=w1006:errorcluster)
                n426 = call "UpdateCurvePar.vi"("error in (no error)"=w1006, "PlotChange"=w1007, "Interface en entrée"=w1004) -> ("error out"=w1005:errorcluster, "Interface en sortie"=w1003:refnum<class "Interface.lvclass">)  [unwired: 7 in]
              }
              frame "Goto2DGraphPos" {
                n427 = local read "Acq"() -> (w1011:bool)
                n428 = case shown="Faux" w1011 {
                  tunnel: w1016 -> [w1025 _]
                  tunnel: w1015 -> [w1024 w1029]
                  tunnel: w1014 -> [w1023 w1028]
                  tunnel: [w1022 w1028] -> w1013
                  tunnel: [w1021 w1029] -> w1012
                  frame False {
                    n429 = Variant To Data(error in=w1024, type=T12 {[], "XparInstrInd"=0, "YparInstrInd"=0} ("cluster"), Variant=w1025) -> (data=w1027:T12, error out=w1017:errorcluster)
                    n430 = Unbundle(w1027) -> (w1026:dbl[], "XparInstrInd"=w1019:i32, "YparInstrInd"=w1018:i32)
                    n431 = call "Send2DGotoComm.vi"("YParInstInd"=w1018, "error in (no error)"=w1017, "XY Data"=w1026, "XParInstInd"=w1019, "Interface en entrée"=w1023) -> ("error out"=w1021:errorcluster, "Interface en sortie"=w1022:refnum<class "Interface.lvclass">)  [unwired: 5 in]
                  }
                  frame True {
                  }
                }
              }
              frame "ClosedGraph" {
                # "Closed graph either by click of close window button sat title bar or in graph menu"
                # "Message Data rarray:\n1st element: GraphNum\n2nd element: FreeFloating (1) or FA_Embedded(0)"
                n432 = Variant To Data(error in=w1043, type=i32[] [], Variant=w1044) -> (data=w1042:i32[], error out=w1037:errorcluster)
                n433 = call "GetGraphVIName.vi"("ErrIn (NoErr)"=w1037, "Interface In"=w1033) -> ("error out"=w1036:errorcluster, "Interface Out"=w1032:refnum<class "Interface.lvclass">, "GraphNumbers"=w1035:i32[])  [unwired: 4 in, 3 out]
                n434 = Index Array(array=w1042) -> (element=w1034:i32)  [unwired: 1 in]
                n435 = Search 1D Array(1D array=w1035, element=w1034) -> (index of element=w1031:i32)  [unwired: 1 in]
                n436 = Build Array(w1031) -> (w1041:i32[])
                n437 = call "CloseFAGraph.vi"("error in (no error)"=w1036, "UpdtGphConf"=TRUE, "GraphIndexArr"=w1041, "Interface en entrée"=w1032) -> ("error out"=w1040:errorcluster, "Interface en sortie"=w1039:refnum<class "Interface.lvclass">)  [unwired: 6 in]
              }
              frame "Closed2DGraph" {
                n438 = Variant To Data(error in=w1050, type=0, Variant=w1051) -> (data=w1045:i32, error out=w1049:errorcluster)
                n439 = call "Close2DGraph.vi"("error in (no error)"=w1049, "GraphIndexArr"=w1045, "Interface en entrée"=w1047) -> ("error out"=w1048:errorcluster, "Interface en sortie"=w1046:refnum<class "Interface.lvclass">)  [unwired: 7 in]
              }
            }
            n440 = local write "Interface.lvclass"(w970) -> ()
          }
          event "AcqEnd": Value Change {
            n441 = event-data() -> ("NewVal"=w1055:bool)  [unwired: 1 in, 5 out]
            n442 = case shown="Vrai" w1055 {
              tunnel: w1053 -> [w1056 w1064]
              tunnel: [w1056 w1080] -> w1054
              frame False {
                # "Ce case ne devrait pas se produire"
              }
              frame True {
                w1081 = string[] ["Save Experiment", "Quitter LabScan", "Config Instruments", "Config Experiment", "Config Interface", "SetupGraphConfig", "SetupCalc", "Paramètres du programme", "Data Bindings"]  # disabled during scan items
                w1077 = string[] []  # enabled during scan Item tags
                # "Vérifie le cluster d'erreur de la boucle d'acquisition"
                # "fin de l'acquisition"
                # "on a terminé un scan"
                n443 = call <vilib>:"Clear Errors.vi"("error in (no error)"=w1064) -> ("error out"=w1063:errorcluster)  [unwired: 5 in, 1 out]
                n444 = control-ref of="Discard"() -> (w1069:refnum<vi>)
                n445 = control-ref of="stop"() -> (w1066:refnum<vi>)
                n446 = local read "Interface.lvclass"() -> (w1076:refnum<class "Interface.lvclass">)
                n447 = Build Array(w1069, w1066) -> (w1067:refnum<vi>[])
                n448 = call-poly <userlib>:"SetCtrlPropGenPol.vi"("Error in"=w1063, "Énum"=T2."Enable", "Controls"=w1067) -> ("Error out"=w1068:errorcluster)  [unwired: 3 in, 1 out]
                n449 = call "IncrCurveInd.vi"("error in (no error)"=w1063, "Interface en entrée"=w1076) -> ("error out"=w1065:errorcluster, "Interface en sortie"=w1060:refnum<class "Interface.lvclass">)  [unwired: 8 in]
                n450 = local read "Exper.lvclass"() -> (w1074:refnum<class "Experiment.lvclass">)
                n451 = local read "AcqComp"() -> (w1058:bool)
                n452 = call "SignalAcqStatus.vi"("error in (no error)"=w1065, "Booléen"=FALSE, "Experiment en entrée"=w1074) -> ("error out"=w1073:errorcluster, "Experiment en sortie"=w1072:refnum<class "Experiment.lvclass">)  [unwired: 7 in]
                n453 = local read "ErrorOutAcq"() -> (w1078:errorcluster)
                n454 = call "EndScan.vi"("error in (no error)"=w1073, "AcqComp"=w1058, "Experiment en entrée"=w1072) -> ("error out"=w1062:errorcluster, "PostScanString"=w1057:string, "Experiment en sortie"=w1071:refnum<class "Experiment.lvclass">)  [unwired: 6 in]
                n455 = Current VI's Menubar() -> (w1082:refnum<k9>)
                n456 = call <userlib>:"GestionMenuGen.vi"("error in"=w1068, "ToDisableItems"=w1077, "ToEnableItems"=w1081, "référence de menu"=w1082) -> ("error Out"=w1079:errorcluster)  [unwired: 7 in]
                n457 = local write "Exper.lvclass"(w1071) -> ()
                n458 = call "PostScanUpdate.vi"("error in (no error)"=w1062, "PostScanString"=w1057, "Interface en entrée"=w1060) -> ("error out"=w1061:errorcluster, "Interface en sortie"=w1059:refnum<class "Interface.lvclass">)  [unwired: 7 in]
                n459 = local write "Interface.lvclass"(w1059) -> ()
                n460 = Merge Errors(w1064, w1078, w1079, w1061) -> (w1080:errorcluster)
              }
            }
          }
          event "Scan Function": Value Change {
            n461 = event-data() -> ("NewVal"=w1088:u16)  [unwired: 1 in, 5 out]
            n462 = local read "Exper.lvclass"() -> (w1087:refnum<class "Experiment.lvclass">)
            n463 = local read "user event out"() -> (w1084:refnum<user-event>)
            n464 = local read "queue out"() -> (w1083:refnum<queue>)
            n465 = call "UpdateScanPan.vi"("MainProgQEvent"=w1084, "MainProgQ"=w1083, "error in (no error)"=w1089, "Function"=w1088, "Experiment en entrée"=w1087) -> ("error out"=w1085:errorcluster, "Experiment en sortie"=w1086:refnum<class "Experiment.lvclass">)  [unwired: 3 in, 2 out]
            n466 = local write "Exper.lvclass"(w1086) -> ()
          }
          event "Listbox": Double Click {
            # "Affiche ou cache les courbes"
            n467 = event-data() -> ("Row"=w1094:i32)  [unwired: 1 in, 1 out]
            n468 = local read "Interface.lvclass"() -> (w1093:refnum<class "Interface.lvclass">)
            n469 = call "SetCurvVisible.vi"("error in (no error)"=w1091, "CurveIndex"=w1094, "Interface en entrée"=w1093) -> ("Error out"=w1090:errorcluster, "Interface Out"=w1092:refnum<class "Interface.lvclass">)  [unwired: 7 in]
            n470 = local write "Interface.lvclass"(w1092) -> ()
          }
          event "Listbox": Key Up {
            n471 = event-data() -> ("ScanCode"=w1097:i16)  [unwired: 1 in, 7 out]
            n472 = case shown="83" w1097 {
              tunnel: w1095 -> [w1098 w1100]
              tunnel: [w1098 w1099] -> w1096
              frame 0, Default {
              }
              frame 83 {
                # "On désire effacer une courbe"
                n473 = local read "Acq"() -> (w1101:bool)
                n474 = case shown="Faux" w1101 {
                  tunnel: w1100 -> [w1103 w1112]
                  tunnel: [w1102 w1112] -> w1099
                  frame False {
                    n475 = property on="Listbox" class="LstDér (strict)"() -> ("Value"=w1104:i32[])  [unwired: 2 in, 2 out]
                    n476 = call "Boîte de dialogue utilisateur2"() -> ("OK"=w1105:bool)  [unwired: 18 in, 1 out]
                    n477 = case shown="Vrai" w1105 {
                      tunnel: w1104 -> [_ w1109]
                      tunnel: w1103 -> [w1106 w1111]
                      tunnel: [w1106 w1110] -> w1102
                      frame False {
                        # "Opération annulé par l'utilisateur"
                      }
                      frame True {
                        # "Supprime la courbe"
                        n478 = local read "Interface.lvclass"() -> (w1108:refnum<class "Interface.lvclass">)
                        n479 = call "DeleteDataM.vi"("error in (no error)"=w1111, "CurveNumbers"=w1109, "Interface en entrée"=w1108) -> ("error out"=w1110:errorcluster, "Interface en sortie"=w1107:refnum<class "Interface.lvclass">)  [unwired: 7 in]
                        n480 = local write "Interface.lvclass"(w1107) -> ()
                      }
                    }
                  }
                  frame True {
                    # "L'acquisition est en cours impossible de\nfaire la supression"
                    n481 = call "Boîte de dialogue utilisateur"() -> ()  [unwired: 18 in, 2 out]
                  }
                }
              }
            }
          }
          event "Ouvrir": Value Change {
            # "on demande l'ouverture du fichier de sauvegarde"
            n482 = event-data() -> ("NewVal"=w1113:bool)  [unwired: 1 in, 5 out]
            n483 = case shown="Vrai" w1113 {
              tunnel: w1115 -> [w1116 w1122]
              tunnel: [w1116 w1121] -> w1114
              frame False {
              }
              frame True {
                # "ouvre le fichier dans notepad"
                # "ouvre une boîte de dialogue fichier\nsi le chemin est incorrecte"
                n484 = Empty String/Path?(string/path="path") -> (empty?=w1124:bool)
                n485 = Not A Number/Path/Refnum?(number/path/refnum="path") -> (NaN/Path/Refnum?=w1125:bool)
                n486 = Or(x=w1124, y=w1125) -> (x .or. y?=w1123:bool)
                n487 = case shown="Vrai" w1123 {
                  tunnel: [w1137 w1143] -> w1126
                  tunnel: [w1138 w1142] -> w1127
                  tunnel: "path" -> [w1138 _]
                  tunnel: [_ w1141] -> _
                  tunnel: [w1137 w1139] -> w1117
                  frame False {
                    w1137 = FALSE ("cancelled")
                  }
                  frame True {
                    n488 = File Dialog(4:"Text File" ("pattern label"), 6:"*.txt" ("pattern")) -> (0:w1140:errorcluster, 1:w1143:bool, 3:w1142:path)  [unwired: 5 in, 1 out]
                    n489 = Unbundle By Name(w1140) -> ("status"=w1139:bool)
                    n490 = call <vilib>:"Clear Errors.vi"("error in (no error)"=w1140) -> ("error out"=w1141:errorcluster)  [unwired: 5 in, 1 out]
                  }
                }
                n491 = local write "Ouvrir"(FALSE ("Ouvrir")) -> ()
                n492 = Or(x=w1126, y=w1117) -> (x .or. y?=w1118:bool)
                n493 = case shown="Faux" w1118 {
                  tunnel: w1127 -> [w1130 _]
                  tunnel: w1122 -> [w1129 w1136]
                  tunnel: [w1128 w1136] -> w1121
                  frame False {
                    n494 = local write "path"(w1130) -> ()
                    n495 = Path To String(path=w1130) -> (string=w1132:string)
                    n496 = Concatenate Strings("notepad" ("command line"), " " ("string"), w1132) -> (w1131:string)
                    n497 = call <vilib>:"System Exec.vi"("wait until completion? (T)"=FALSE, "error in (no error)"=w1129, "command line"=w1131) -> ("error out"=w1128:errorcluster)  [unwired: 5 in, 3 out]
                  }
                  frame True {
                  }
                }
              }
            }
          }
          event "stop": Value Change {
            # "Arrête le programme"
            n498 = event-data() -> ("NewVal"=w1146:bool)  [unwired: 1 in]
            n499 = case shown="Vrai" w1146 {
              tunnel: [_ w1160] -> w1149
              tunnel: w1148 -> [w1150 w1157]
              tunnel: [w1150 w1154] -> w1147
              frame False {
              }
              frame True {
                n500 = local read "Experiment Path"() -> (w1153:path)
                n501 = local read "Interface.lvclass"() -> (w1159:refnum<class "Interface.lvclass">)
                n502 = call "SaveInterfSetup.vi"("error in (no error)"=w1157, "Experiment Path"=w1153, "Interface en entrée"=w1159) -> ("error out"=w1156:errorcluster, "Cancel Close Out"=w1152:bool, "SavePath"=w1155:path, "Interface en sortie"=w1158:refnum<class "Interface.lvclass">)  [unwired: 5 in]
                n503 = case shown="Faux" w1152 {
                  tunnel: [TRUE FALSE] -> w1160
                  tunnel: w1158 -> [w1174 _]
                  tunnel: w1156 -> [w1173 w1181]
                  tunnel: w1155 -> [w1171 _]
                  tunnel: [w1165 w1181] -> w1154
                  tunnel: [_ FALSE ("stop")] -> w1151
                  frame False {
                    n504 = local read "Exper.lvclass"() -> (w1177:refnum<class "Experiment.lvclass">)
                    n505 = local read "queue out"() -> (w1167:refnum<queue>)
                    n506 = local read "user event out"() -> (w1164:refnum<user-event>)
                    n507 = call "UnloadExp.vi"("error in (no error)"=w1173, "Experiment en entrée"=w1177) -> ("error out"=w1175:errorcluster, "Experiment en sortie"=w1176:refnum<class "Experiment.lvclass">)  [unwired: 7 in, 1 out]
                    n508 = call "SaveExpConfig.vi"("error in (no error)"=w1175, "Experiment"=w1171, "Experiment.lvclass"=w1176) -> ("error out"=w1172:errorcluster)  [unwired: 7 in, 1 out]
                    n509 = call "UnloadInterface.vi"("Interface en entrée"=w1174, "error in (no error)"=w1172) -> ("ListBoxRef"=w1170:refnum<vi>, "error out"=w1168:errorcluster)  [unwired: 6 in, 6 out]
                    n510 = call-poly <userlib>:"SetCtrlPropGenPol.vi"("Error in"=w1168, "Énum"=T2."ReinitToDefVal", "Controls"=w1170) -> ("Error out"=w1163:errorcluster)  [unwired: 3 in, 1 out]
                    n511 = Release Queue(queue=w1167, force destroy? (F)=TRUE, error in (no error)=w1163) -> (error out=w1161:errorcluster)  [unwired: 2 out]
                    n512 = Destroy User Event(user event=w1164, error in=w1163) -> (error out=w1162:errorcluster)
                    n513 = Merge Errors(w1163, w1161, w1162) -> (w1165:errorcluster)
                  }
                  frame True {
                  }
                }
                n514 = local write "stop"(w1151) -> ()
              }
            }
          }
        }
      }
      n515 = while {
        shift-right: [w1184] -> _
        shift-left: w137 -> [w1185]
        shift-left: w137 -> [w1183]
        stop <- "stop" stop-if-true
        # "Boucle d'acquisition"
        n516 = local read "sem1"() -> (w1182:T1)
        n517 = case shown="Vrai" w1185 {
          tunnel: errorcluster {"status"=FALSE, "code"=0, "source"=""} ("error in") -> [w1191 w1226]
          tunnel: [w1195 FALSE] -> w1184
          tunnel: w1183 -> [w1194 _]
          tunnel: w1182 -> [w1188 w1212]
          frame False {
            # "lit le bouton aquisition"
            # "L'acquisition est arrêtée"
            n518 = call <vilib>:"Acquire Semaphore.vi"("error in (no error)"=w1191, "semaphore"=w1188) -> ("error out"=w1190:errorcluster, "semaphore out"=w1189:T1)  [unwired: 3 in, 1 out]
            n519 = case shown="Vrai" w1194 {
              tunnel: w1189 -> [w1200 w1202]
              tunnel: [w1200 w1202] -> w1192
              tunnel: [w1199 w1203] -> w1193
              tunnel: w1190 -> [w1199 w1203]
              frame False {
                # "L'acquisition est arrêté\nRien à faire dans ce cas"
              }
              frame True {
                # "Réinitialise la variable d'arrêt"
                # "on signale la fin de l'acquisition à la boucle d'évènement"
                # "on sort d'une acquisition"
                n520 = local write "AcqStop"(FALSE ("Acq")) -> ()
                n521 = property on="AcqEnd" class="Bool (strict)"("Valeur (Signalisation)"=TRUE) -> ()  [unwired: 2 in, 2 out]
                n522 = local write "Acq"(FALSE ("Acq")) -> ()
              }
            }
            n523 = Wait (ms)(milliseconds to wait=u32 200) -> ()  [unwired: 1 out]
            n524 = flat-sequence {
              tunnel: w1192 -> [w1207]
              tunnel: w1193 -> [w1208]
              tunnel: [w1208] -> w1197
              tunnel: [w1207] -> w1196
              tunnel: ["Acq"] -> w1195
              frame #0 {
              }
            }
            n525 = call <vilib>:"Release Semaphore.vi"("error in (no error)"=w1197, "semaphore"=w1196) -> ()  [unwired: 4 in, 2 out]
          }
          frame True {
            # "(nb point)^^"
            # "nb pos. par courbe>>"
            # "(nb point-1)^^"
            # "Une Acquisition est en cours"
            n526 = local read "Scan Function"() -> (w1210:u16)
            n527 = local read "Exper.lvclass"() -> (w1221:refnum<class "Experiment.lvclass">)
            n528 = local read "Single Par"() -> (w1209:bool)
            n529 = local read "Interface.lvclass"() -> (w1214:refnum<class "Interface.lvclass">)
            n530 = Decrement(x="nb pos") -> (x-1=w1220:i32)
            n531 = Tick Count (ms)() -> (millisecond timer value=w1217:u32)
            n532 = while {
              tunnel: w1220 -> [w1288]
              shift-right: [w1270] -> w1218
              shift-left: w1226 -> [w1275]
              tunnel: w1212 -> [w1283]
              tunnel: "nb pos" -> [w1285]
              tunnel: [w1279] -> w1219
              tunnel: [w1278] -> w1223
              tunnel: w1217 -> [w1277]
              tunnel: "DataFileRef" -> [w1276]
              shift-right: [w1265] -> w1215
              shift-left: w1221 -> [w1274]
              shift-right: [w1271] -> w1213
              shift-left: w1214 -> [w1247]
              tunnel: w1210 -> [w1252]
              tunnel: w1209 -> [w1251]
              i -> [w1246]
              stop <- w1293 stop-if-true
              # "Nb point restant"
              # "R:Index du point en cours"
              # "IQ:Index de la courbe en cours"
              # "7.Vérifie si on a acq. tous les points"
              n533 = call "Scan.vi"("Function"=w1252, "error in (no error)"=w1275, "Single"=w1251, "Index"=w1246, "ExperimentIn"=w1274) -> ("error out"=w1242:errorcluster, "TimesArray"=→"ScanTimes":u32[], "ScanParsOut"=w1256:dbl[], "ExperimentOut"=w1273:refnum<class "Experiment.lvclass">)  [unwired: 3 in]
              n534 = call <userlib>:"T_At_Wire_Err.vi"("error in (no error)"=w1242) -> ("Clock(ms)"=w1238:u32, "error out"=w1241:errorcluster)  [unwired: 8 in, 1 out]
              n535 = call "Measure.vi"("error in"=w1241, "Scan"=TRUE, "IndicePoint"=w1246, "Experiment.lvclass In"=w1273) -> ("error out"=w1240:errorcluster, "ArrDevDat"=w1245:T17[], "Données"=w1257:dbl[], "Experiment.lvclass Out"=w1249:refnum<class "Experiment.lvclass">, "SaveArrVarPar"=w1244:bool[], "MeasTimes"=→"MeasTimes":u32[])  [unwired: 2 in]
              n536 = Greater Or Equal?(x=w1246, y=w1288) -> (x >= y?=w1278:bool)
              n537 = Subtract(x=w1285, y=w1246) -> (x-y=w1287:i32)
              n538 = call <userlib>:"T_At_Wire_Err.vi"("InitClock(ms)"=w1238, "error in (no error)"=w1240) -> ("Clock(ms)"=w1235:u32, "error out"=w1239:errorcluster, "Delta(ms)"=→"MeasTime":u32)  [unwired: 7 in]
              n539 = call "AddCurveArrDev.vi"("SaveArrVarPar"=w1244, "ArrDevDat"=w1245, "error in"=w1239, "CurPointInd"=w1246, "Exper.lvclass In"=w1249, "InterfaceIn"=w1247) -> ("error out"=w1250:errorcluster, "InterfaceOut"=w1248:refnum<class "Interface.lvclass">)  [unwired: 4 in]
              n540 = call "WriteDataQ.vi"("IndPoint"=w1246, "error in (no error)"=w1250, "DataIn"=w1257, "ScanParIn"=w1256, "Interface en entrée"=w1248) -> ("error out"=w1266:errorcluster, "CrvIndex"=w1253:i32, "CurCrvPointInd"=w1254:i32, "Interface en sortie"=w1263:refnum<class "Interface.lvclass">)  [unwired: 3 in]
              n541 = Build Array (concatenate)(w1256, w1257) -> (w1272:dbl[])
              n542 = To Unsigned Long Integer(number=w1287) -> (unsigned 32bit integer=w1282:u32)
              "Points Left" <- w1282
              n543 = call "Calculate.vi"("error in"=w1266, "IndicePoint"=w1246, "Experiment.lvclass In"=w1249) -> ("error out"=w1261:errorcluster, "Données"=w1255:dbl[], "Experiment.lvclass Out"=w1265:refnum<class "Experiment.lvclass">)  [unwired: 6 in]
              n544 = Build Array (concatenate)(w1272, w1255) -> (w1264:dbl[])
              n545 = call "WriteCalcDatQ.vi"("DataIn"=w1255, "error in (no error)"=w1261, "CrvIndexIn"=w1253, "CurCrvPointIndIn"=w1254, "Interface en entrée"=w1263) -> ("error out"=w1260:errorcluster, "CrvIndex"=w1258:i32, "CurCrvPointInd"=w1259:i32, "Interface en sortie"=w1262:refnum<class "Interface.lvclass">)  [unwired: 3 in]
              n546 = call "Refresh2DGraph.vi"("Data"=w1257, "error in (no error)"=w1260, "CurveIndex"=w1258, "PointIndex"=w1259, "Interface en entrée"=w1262) -> ("error out"=w1236:errorcluster, "Interface en sortie"=w1269:refnum<class "Interface.lvclass">)  [unwired: 5 in]
              n547 = call "DataWriteTxt.vi"("DataFileRef"=w1276, "NewDataIn"=w1264, "error in (no error)"=w1261) -> ("error out"=w1270:errorcluster)  [unwired: 10 in, 2 out]
              n548 = call <userlib>:"T_At_Wire_Err.vi"("InitClock(ms)"=w1235, "error in (no error)"=w1236) -> ("Clock(ms)"=w1230:u32, "error out"=w1233:errorcluster, "Delta(ms)"=→"WrtDatDel":u32)  [unwired: 7 in]
              n549 = call "RefreshGraphArr.vi"("error in (no error)"=w1233, "Interface en entrée"=w1269) -> ("error out"=w1232:errorcluster, "Interface en sortie"=w1271:refnum<class "Interface.lvclass">)  [unwired: 8 in]
              n550 = flat-sequence {
                tunnel: [w1294] -> w1284
                tunnel: w1292 -> [w1296]
                tunnel: [w1296] -> w1291
                tunnel: w1290 -> [w1295]
                tunnel: [w1295] -> w1289
                frame #0 {
                  n551 = local read "AcqStop"() -> (w1294:bool)
                }
              }
              n552 = call <userlib>:"T_At_Wire_Err.vi"("InitClock(ms)"=w1230, "error in (no error)"=w1232) -> ("error out"=w1231:errorcluster, "Delta(ms)"=→"WrtGrpDel":u32)  [unwired: 7 in, 1 out]
              n553 = call <vilib>:"Acquire Semaphore.vi"("error in (no error)"=w1231, "semaphore"=w1283) -> ("error out"=w1290:errorcluster, "semaphore out"=w1292:T1)  [unwired: 3 in, 1 out]
              n554 = Unbundle By Name(w1231) -> ("status"=w1286:bool)
              n555 = call "TempsÉcouléGen.vi"("error in (no error)"=w1231, "Points effectués"=w1246, "Points restant"=w1282, "Temps initiale"=w1277) -> ("error out"=w1280:errorcluster, "Temps Restant"=→"Temps Balayage":dbl, "AvgPointTime(ms)"=→"AvgPointTime(ms)":u32)  [unwired: 3 in, 2 out]
              n556 = call <vilib>:"Release Semaphore.vi"("error in (no error)"=w1289, "semaphore"=w1291) -> ("error out"=w1281:errorcluster)  [unwired: 4 in, 1 out]
              n557 = Compound Arithmetic op=OR(w1284, w1286, w1278) -> (w1293:bool)
              n558 = Merge Errors(w1280, w1281) -> (w1279:errorcluster)
            }
            "AcqComp" <- w1223
            n559 = call <vilib>:"Clear Errors.vi"("error in (no error)"=w1219) -> ("error out"=w1216:errorcluster)  [unwired: 5 in, 1 out]
            n560 = local write "Exper.lvclass"(w1215) -> ()
            n561 = local write "Interface.lvclass"(w1213) -> ()
            n562 = Merge Errors(w1218, w1216) -> (→"ErrorOutAcq":errorcluster)
          }
        }
      }
      n563 = Not(x=w139) -> (.not. x?=w136:bool)
    }
  }
  n564 = local write "stop"(w13) -> ()
  "error out" <- w10
